vi "IV_Sweep_tool_Probe_Station_Resistance_2PP_2019_11_20.vi"() -> ()   [LabVIEW 2017]
doc: "I. Description:\nThis example demonstrates how to continuously acquire and generate data at the same time, synchronized with one another.\n\nII. Instructions for Running:\n1. Select the physical channel to correspond to where your signal is input on the DAQ device. Also, select the corresponding channel for where your signal is being generated.\n2. Enter the minimum and maximum voltage ranges.\nNote: For better accuracy try to match the input range to the expected voltage level of the measured signal.\n3. Set the sample rate of the acquisition.\nNote: The rate should be at least twice as fast as the maximum frequency component of the signal being acquired. \n6. Select the Rate for the generation\n7. Select what type of signal to generate and the amplitude.\nNote: This example requires two DMA channels to run. If your hardware does not support two DMA channels, you need to set the Data Transfer Mechanism property for the Analog Output Task to use \"Interrupts\". The Data Transfer Mechanism property is located in the DAQmx Channel Property hierarchy at:\n\nDAQmx Channel Property Node>>Analog Output>>General Properties>>Advanced>>Data Transfer and Memory>>Data Transfer Mechanism\n\nRefer to your device documentation to determine how many DMA channels are supported for your hardware.\n\nIII. Block Diagram Steps:\n1. Create an analog input voltage channel. Also, create an analog output voltage channel.\n2. Set the rate for the sample clock. Additionally, define the sample mode to be continuous. Also, set the sample clock rate for the signal generation.\n2a. Call the Get Terminal Name with Device Prefix VI. This will take a Task and a terminal and create a properly formatted device + terminal name to use as the source of the Trigger.\n3. Define the parameters for a Digital Edge Start Trigger. Set the Analog output to trigger off the AI Start Trigger. This is an internal trigger signal.\n4. Use the Basic Function Generator VI to create the signal to be generated.\n5. Call the Start VI to arm the two functions. Make sure the analog output is armed before the analog input. This will ensure both will start at the same time.\n6. Read the waveform data in a loop until the user hits the stop button or an error occurs. The Is Task Done? VI is used to check for errors in the Analog Output Task.\n7. Call the Clear VI to Clear the Task\n8. Use the popup dialog box to display an error if any.\n\nIV. I/O Connections Overview:\nMake sure your signal input/output terminals match the Physical Channel I/O controls."
uses:
  <vilib>/Utility/error.llb/DialogType.ctl
  <vilib>/DAQmx/write.llb/DAQmx Write (Analog 2D DBL NChan NSamp).vi
  <vilib>/DAQmx/read.llb/DAQmx Read (Analog 1D DBL NChan 1Samp).vi
  <vilib>/DAQmx/write.llb/DAQmx Write (Analog DBL 1Chan 1Samp).vi
  <vilib>/DAQmx/read.llb/DAQmx Read (Analog DBL 1Chan 1Samp).vi
  <vilib>/Analysis/baseanly.llb/Mean (DBL).vi
  <vilib>/DAQmx/write.llb/DAQmx Write (Analog 1D DBL NChan 1Samp).vi
  <vilib>/DAQmx/create/channels.llb/DAQmx Create Channel (AO-Voltage-Basic).vi
  <vilib>/DAQmx/create/channels.llb/DAQmx Create Channel (AI-Voltage-Basic).vi
  <vilib>/DAQmx/configure/timing.llb/DAQmx Timing (Sample Clock).vi
  <vilib>/DAQmx/configure/trigger.llb/DAQmx Start Trigger (Digital Edge).vi
  <vilib>/DAQmx/miscellaneous.llb/DAQmx Fill In Error Info.vi
  <vilib>/Utility/file.llb/Write To Spreadsheet File (DBL).vi
  <vilib>/Utility/file.llb/Write To Spreadsheet File (string).vi
  pid/pid.llb/PID (DBL).vi
  pid/pid.llb/PID Output Rate Limiter (DBL).vi
  <vilib>/ptbypt/NI_PtbyPt.lvlib
  <resource>/objmgr/daqmx.rc
  <vilib>/Analysis/NI_AALBase.lvlib
  <vilib>/Analysis/NI_AALPro.lvlib
panel:
  in  "Take a Screenshot":bool=TRUE
  in  "Current Amplifier\n1/Gain  (A/V)":dbl=-1e-11 format="%#_13g"
  out "Date and Time":string
  out "Bias Sweep 2":dbl[](graph)
  out "Array":dbl[](array[numeric])
  out "intercept":dbl
  out "Resistance (Ohms) \n[AI 1 must be connected to Vout (AO 0)]\n[Ensure current amplifier gain is correct]":dbl
  out "RTD-IV":cluster{dbl[], dbl[]}(graph)
  in  "Bias Offset Correct":dbl
  out "Bias Sweep":dbl[](graph)
  out "element":dbl
  out "mean":dbl format="%.6f"
  out "size(s)":i32
  out "Numeric":i32
  in  "PID":bool=TRUE caption="Step Z"
  in  "Tab Control":enum32{"PID Controller", "Tapping Controls"}(tab)=enum."Tapping Controls"
  in  "Proportional Gain":dbl=0.0001
  in  "Integral Gain":dbl=1e-07
  in  "Differential Gain":dbl=1e-05
  in  "Setpoint":dbl=0.1
  in  "Piezo Delta rate":dbl=1000.0
  in  "Min Current":dbl=0.002
  in  "Max Current":dbl=10.2
  in  "Ramp Rate":dbl=20.0
  in  "Make Contact":i32=1200
  in  "Break Contact":i32=500
  in  "Step Length":i32=100
  in  "Step Max":dbl=0.3
  in  "Step Min":dbl=0.05
  out "Tapping Stop":bool
  out "Case":i32
  in  "Contact Cycles":i32
  in  "Tapping":bool caption="Step Z"
  out "x/y":dbl
  out "Waveform Chart":dbl(graph)
  in  "Analog Output 1":dbl(slide) min=-10.0 max=10.0 step=0.001 scale=-10.0..10.0
  in  "Manual Z":bool caption="Step Z"
  in  "Sweep Amplitude":dbl=10.0
  in  "Stop Sweep":bool
  out "Connections 2":string="AI0=Current\nAI1=Bias\nAI2=dI/dV\nAI3=d2I/dV2\nAI4=X-Axis\nAI5=Z-Axis\n"
  out "Connections":string="AO0=Bias\nAO1=Z-axis\nAO2=X-Axis\nAO3=NA"
  out "Save Indicator":bool
  in  "Z-Direction":bool caption="Step Z"
  in  "Update Bias":bool
  in  "Save IV":bool
  in  "Save Decay":bool
  in  "Sweep Bias":bool
  in  "Step Z":bool
  in  "Comments and Experimental Notes":string="Molecule=TP4\nGain=10nA\nBias Gain=div/1\nSweep Freq.=0.0008Hz\nRef. Bias=4mV\nRef. Freq=2.977kHz\nGain LIA1=2mV\nTC LIA1=1s\nGain LIA2=5mV\nTC LIA2=1s\nLIA1=EGG\nLIA2=SRS\nEGG is driving(possible 5mV offset)"
  in  "Filenumber":i32
  in  "DATA Filename":string="Data_"
  in  "Data Directory":path=path "E:/Research/Data"
  out "Current Decay":cluster{dbl[], dbl[]}(graph)
  out "d2I/dV2":cluster{dbl[], dbl[]}(graph)
  out "dI/dV":cluster{dbl[], dbl[]}(graph)
  out "IV":cluster{dbl[], dbl[]}(graph)
  in  "# Samples":i32=2000
  in  "Frequency (Hz)":dbl=0.1
  out "Measurement 2":cluster{i32, dbl, dbl[]}(graph) caption="Measurement"
  out "Actual Update Generation Rate 2":dbl=5000.0 caption="Actual Update Generation Rate" format="%0.2f"
  in  "stop 3":bool
  in  "Bias":dbl caption="Bias Start Point" step=0.1 format="%_3g"
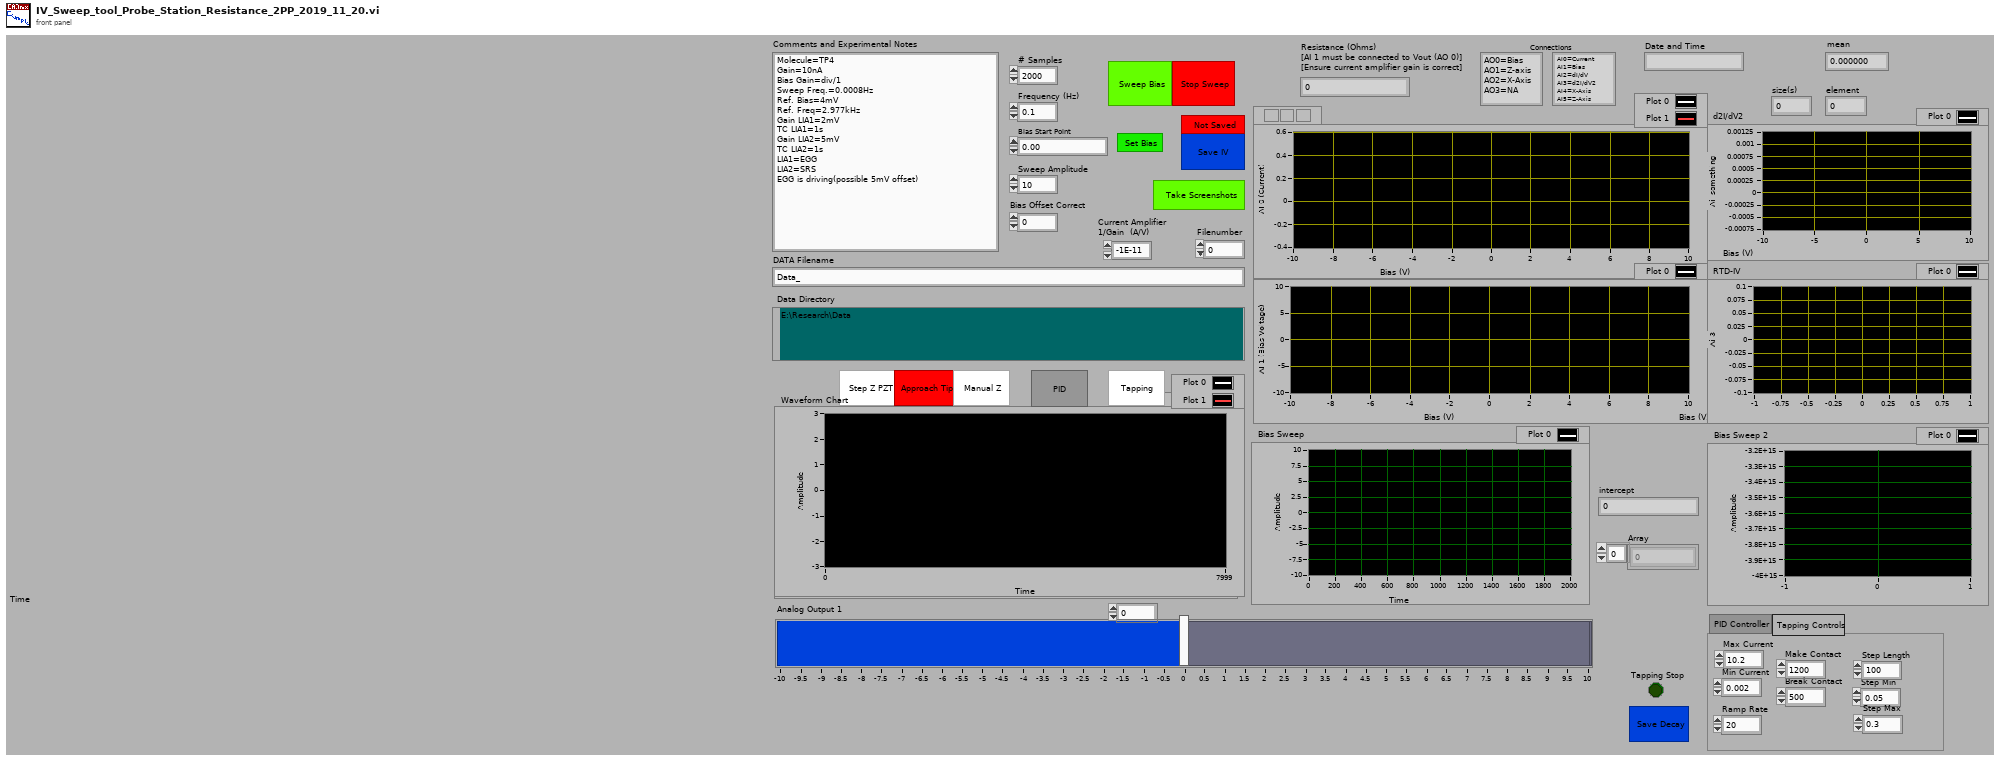
[diagram p1: front panel]
types:
  T1 = enum16{"open", "replace", "create", "open or create", "replace or create", "replace or create with confirmation"}
  T2 = typedef "DialogType.ctl" = u16
  T3 = cluster{"Proportional Gain":dbl, "Integral Gain ":dbl, "Differential Gain":dbl}
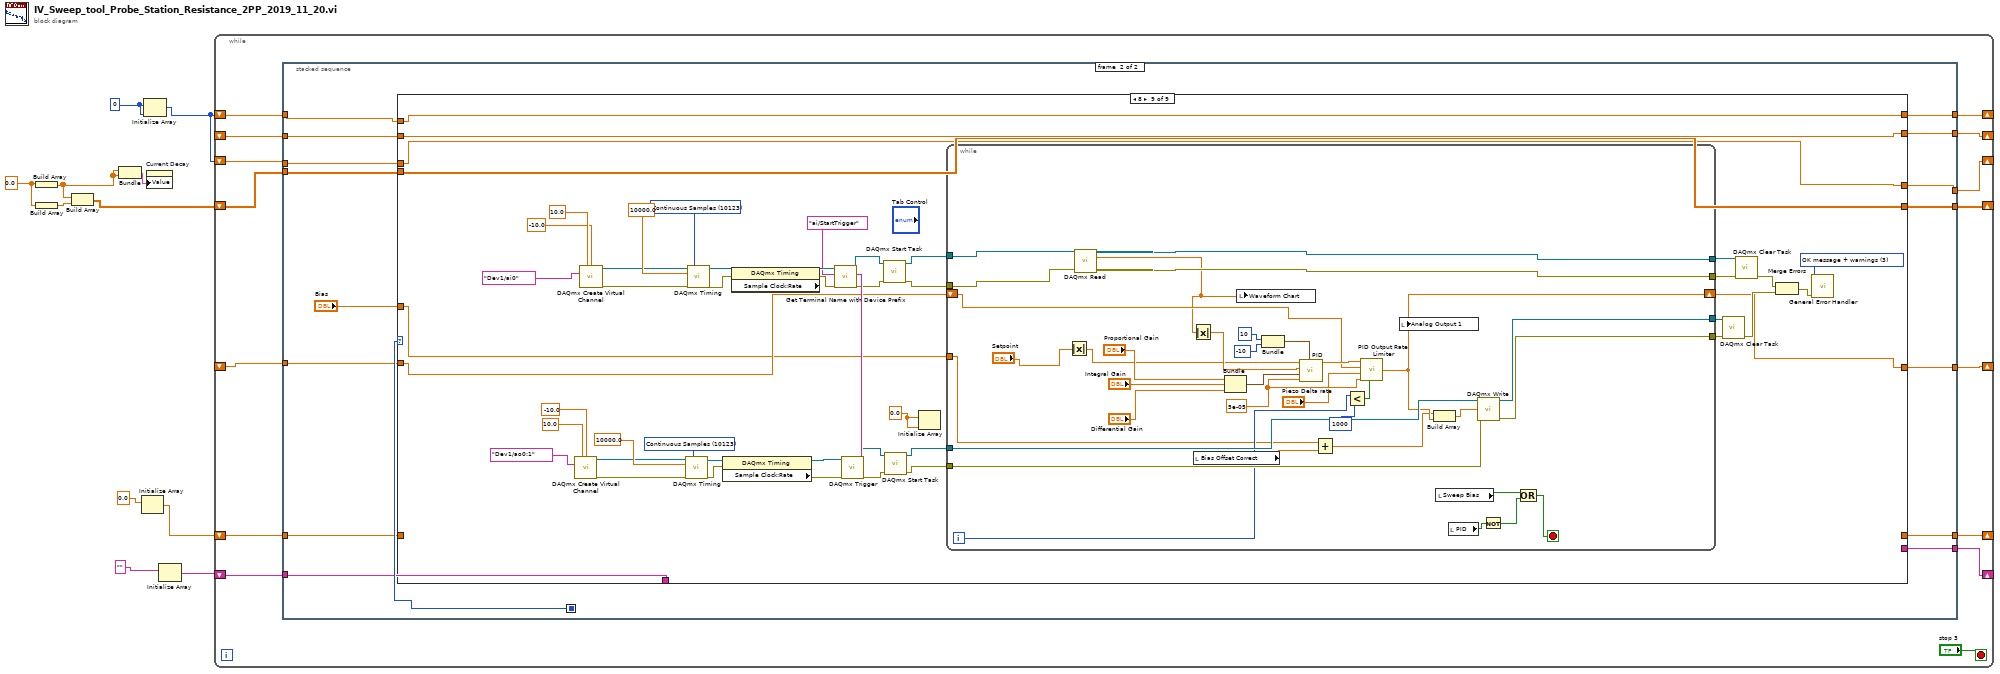
[diagram p0: block diagram]
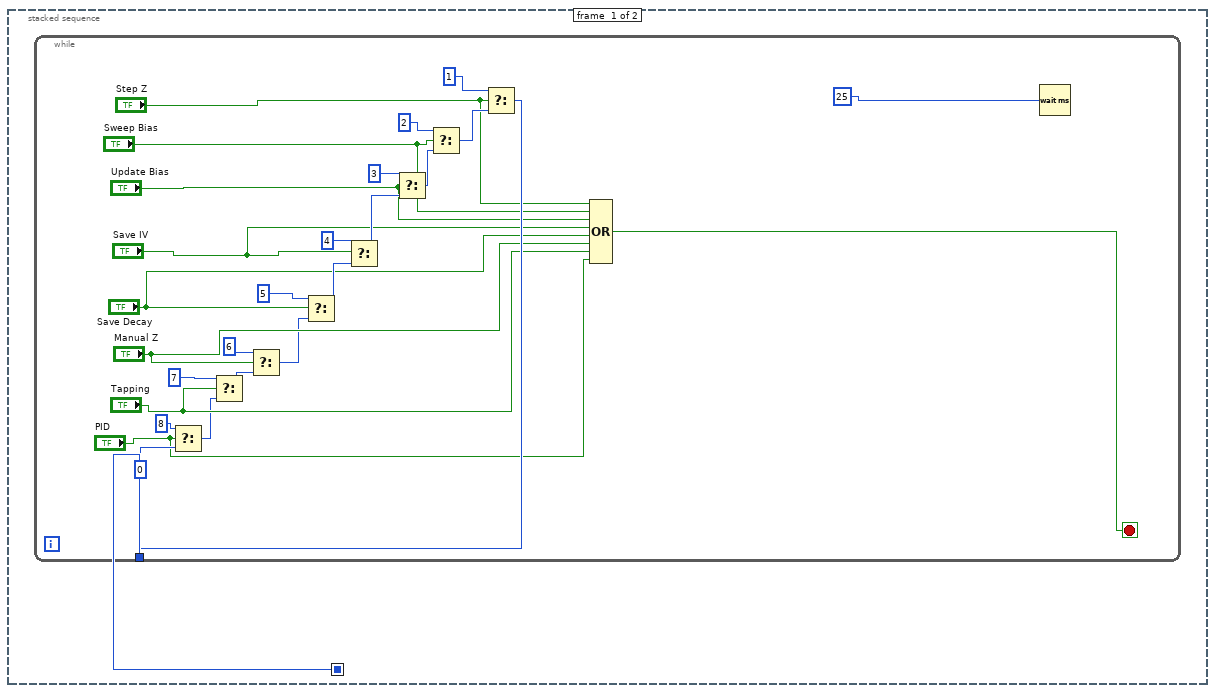
[diagram p2: hidden frame]
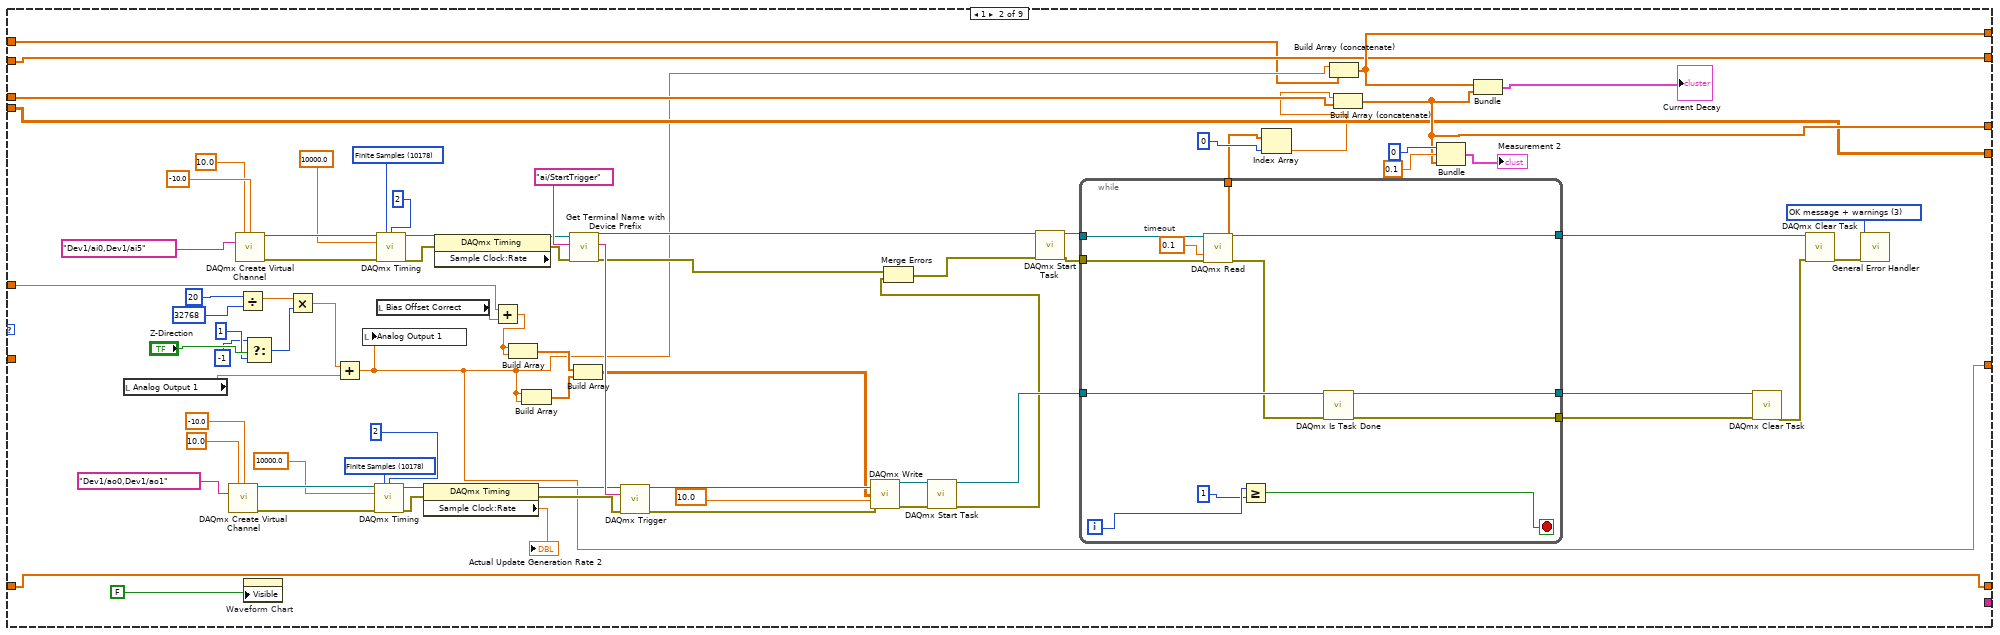
[diagram p4: hidden frame]
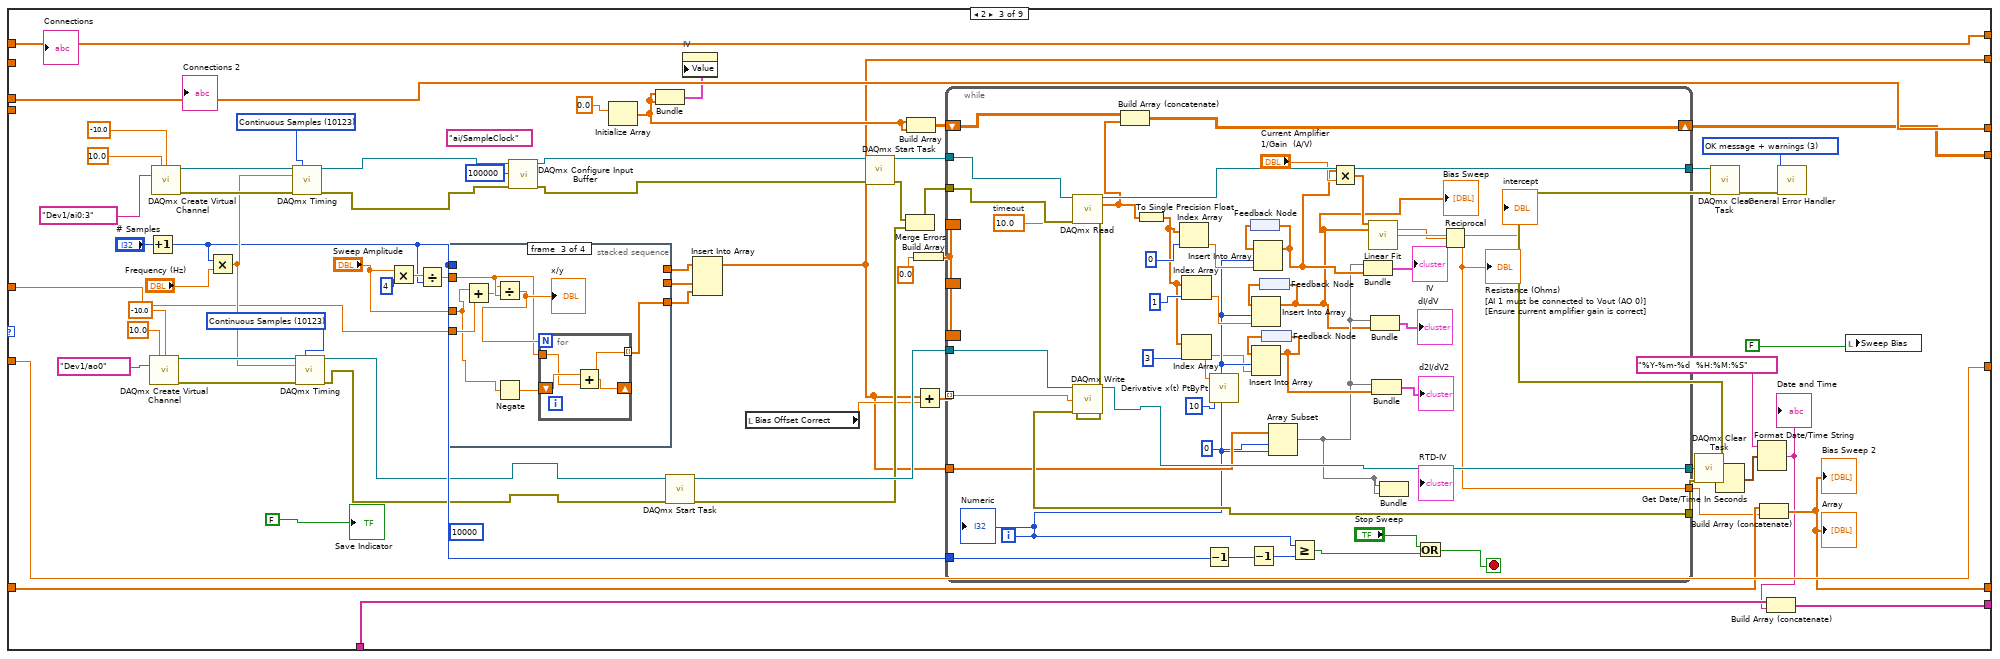
[diagram p5: hidden frame]
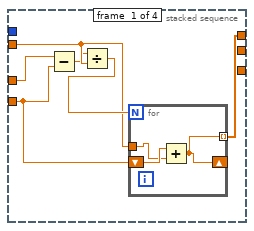
[diagram p6: hidden frame]
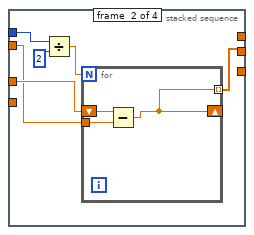
[diagram p7: hidden frame]
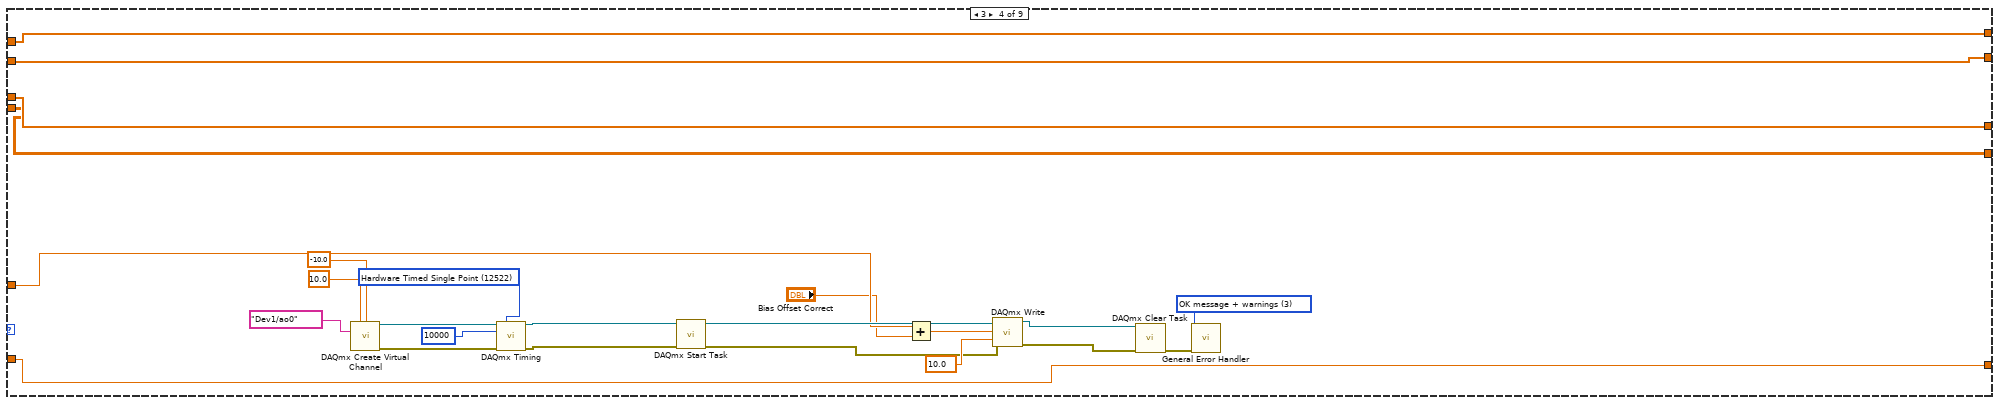
[diagram p9: hidden frame]
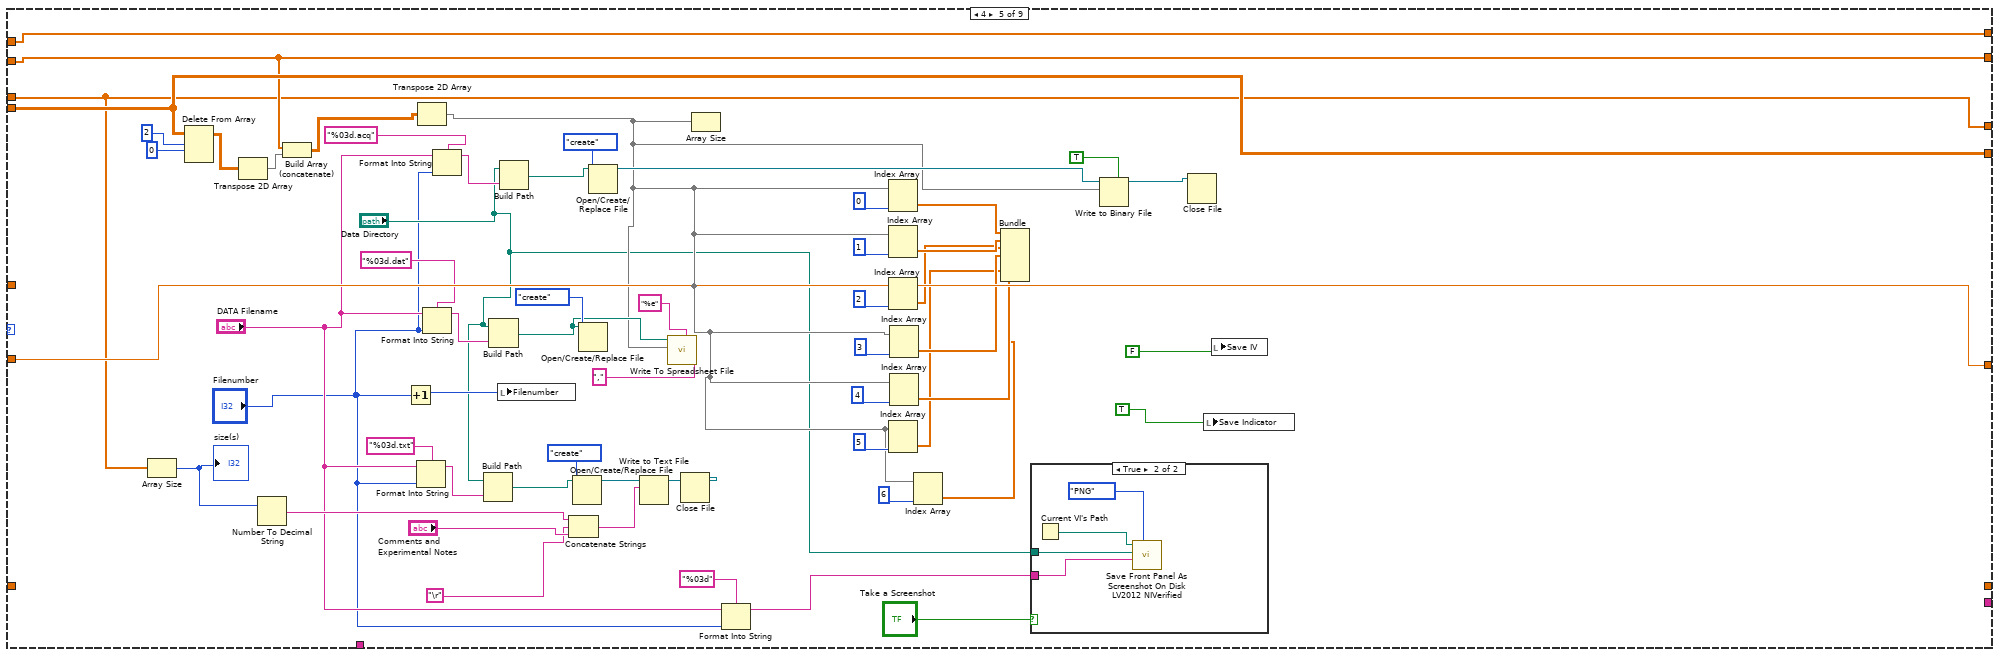
[diagram p10: hidden frame]
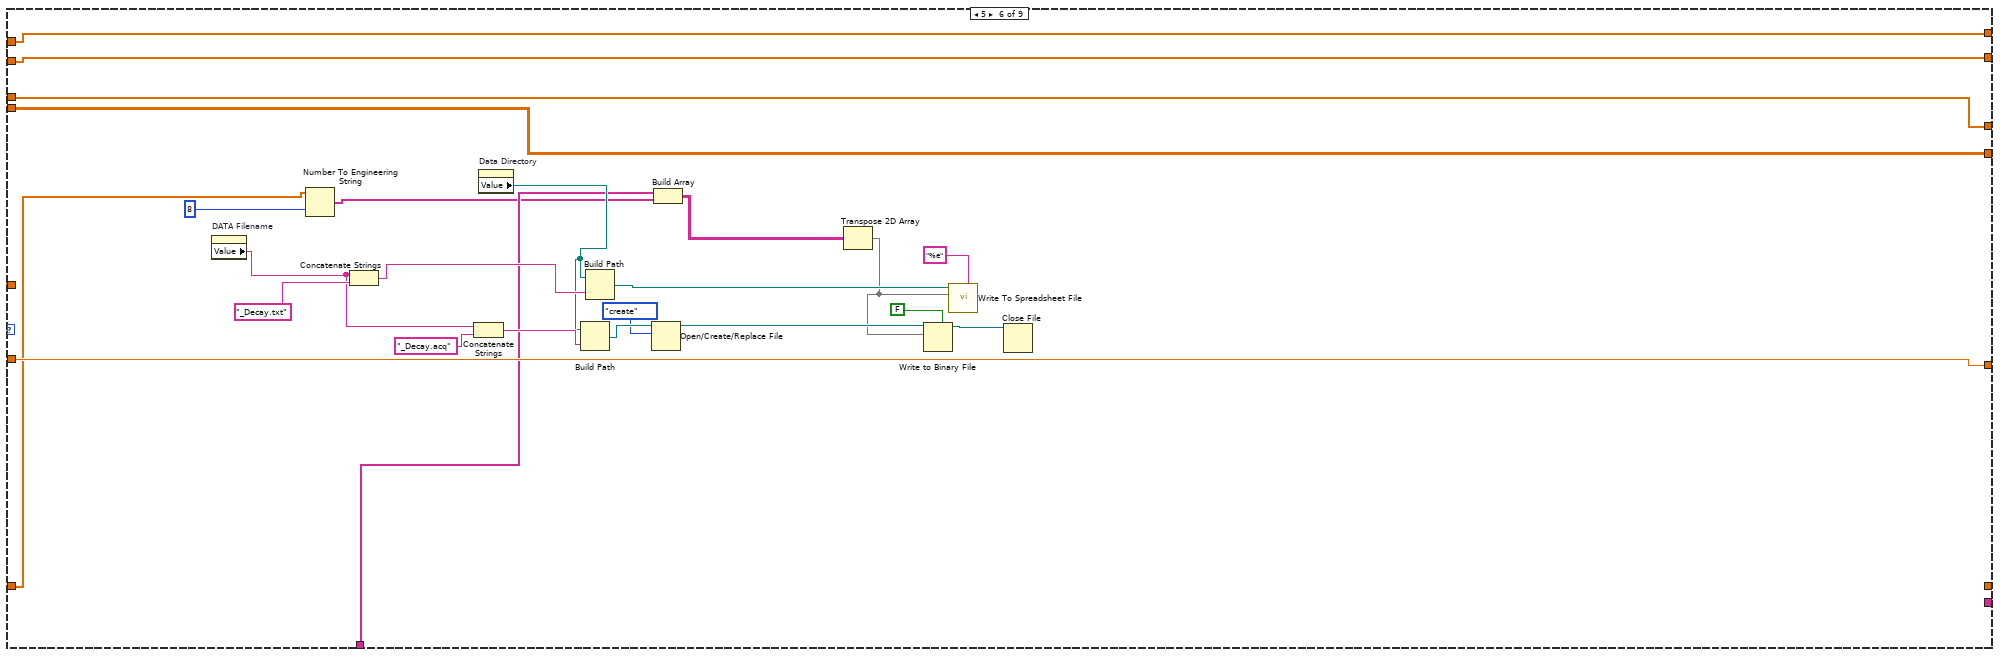
[diagram p12: hidden frame]
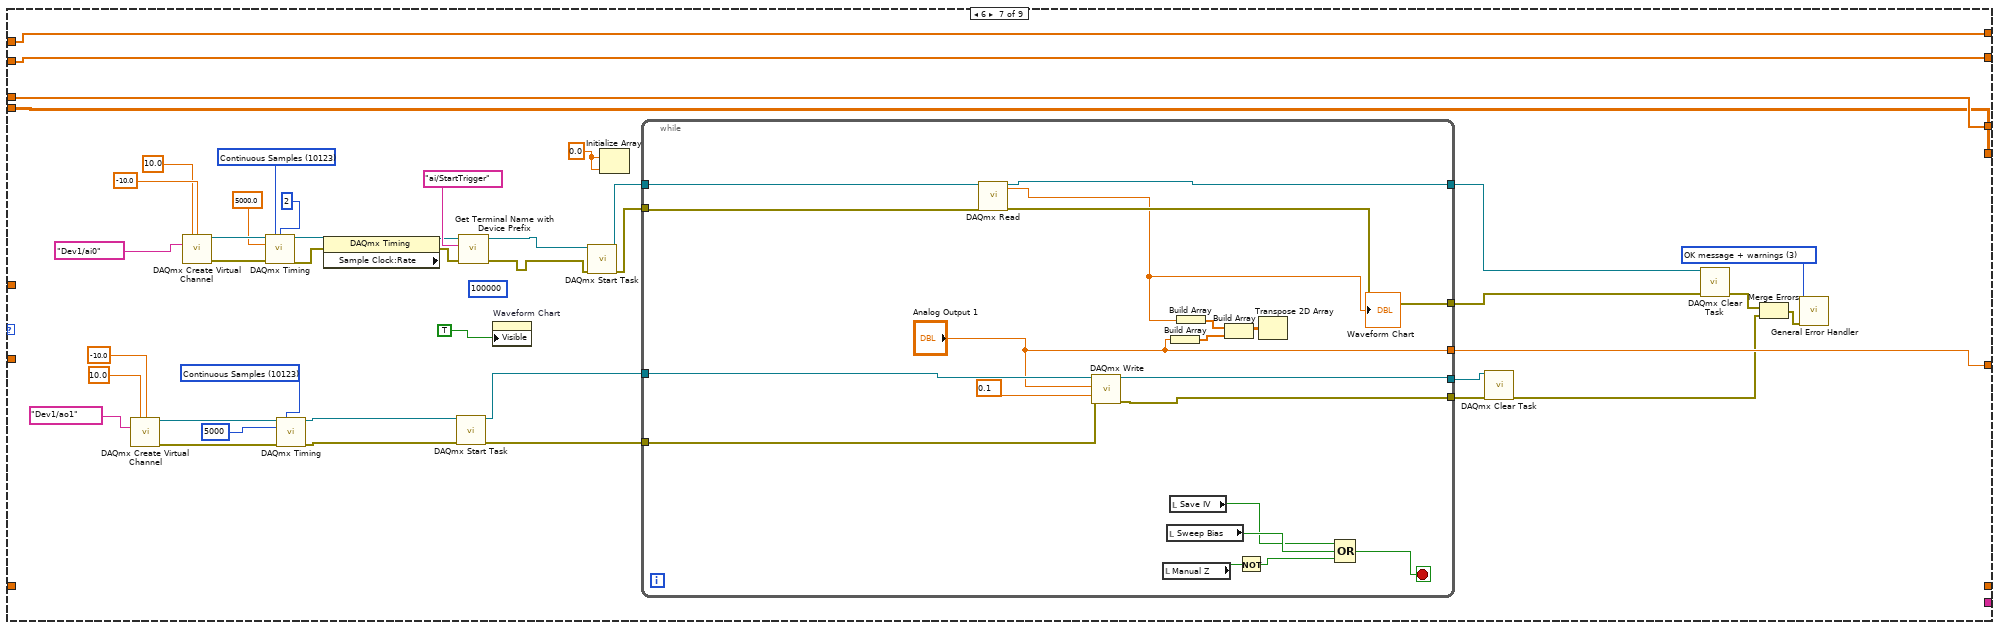
[diagram p13: hidden frame]
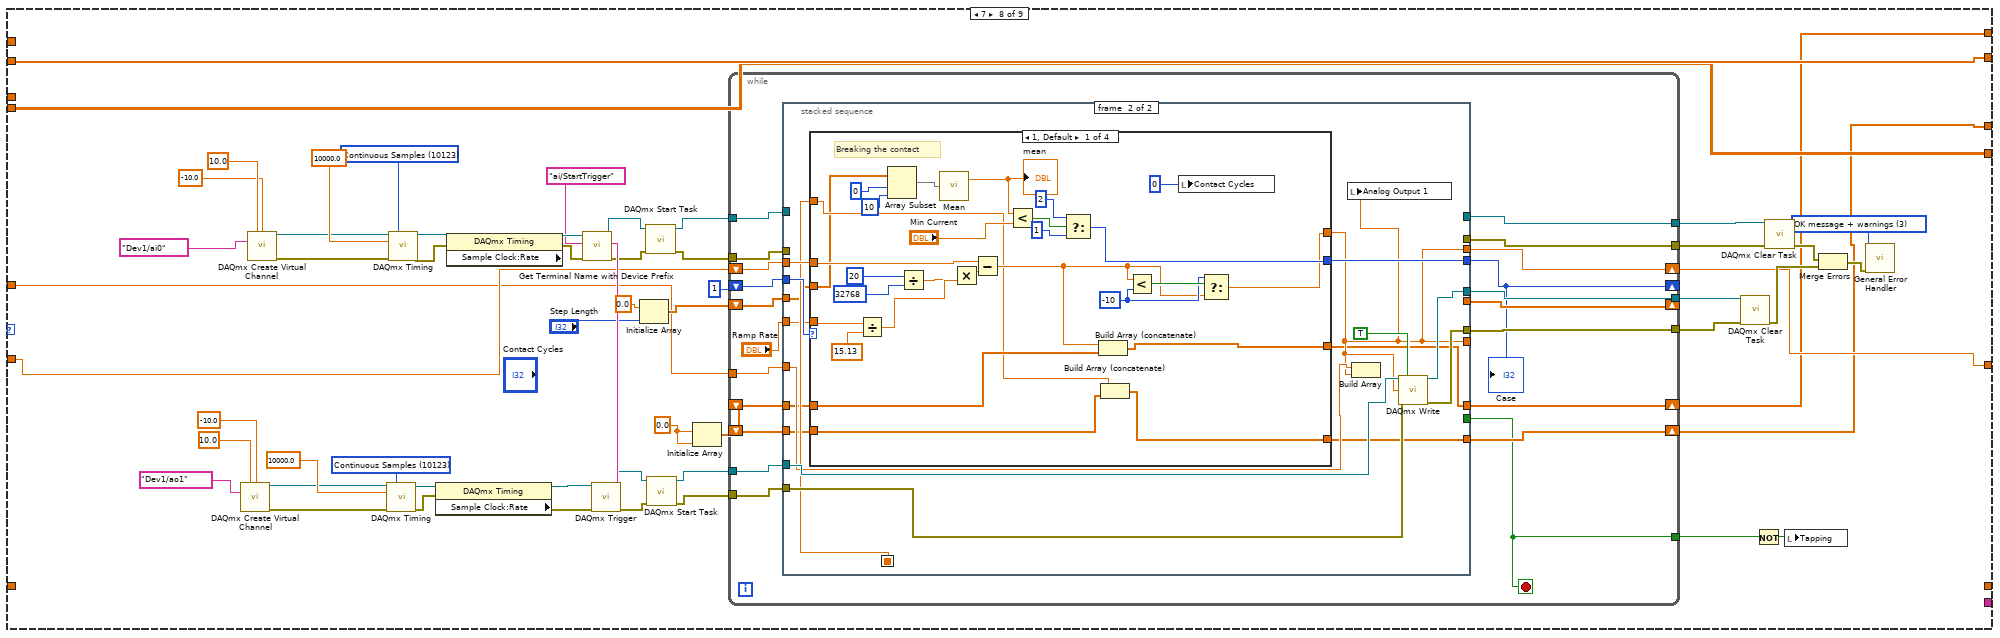
[diagram p14: hidden frame]
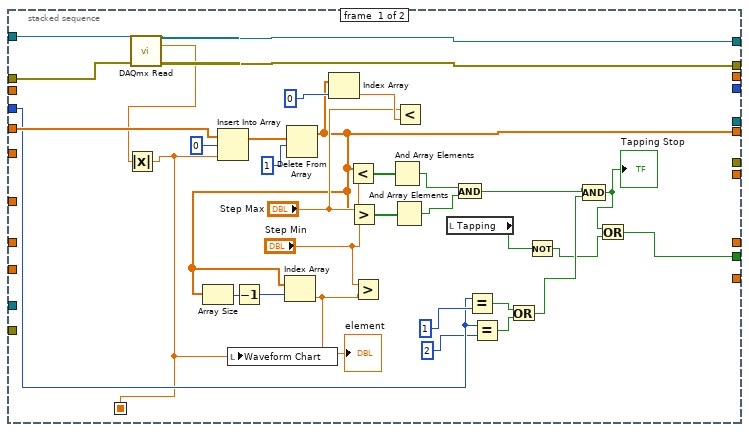
[diagram p15: hidden frame]
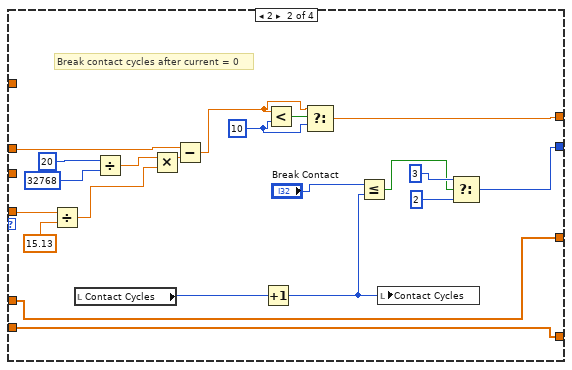
[diagram p16: hidden frame]
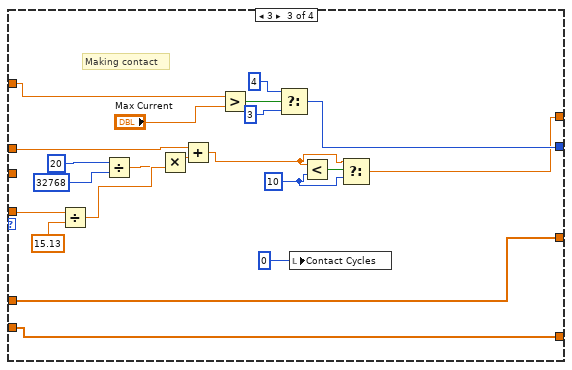
[diagram p17: hidden frame]
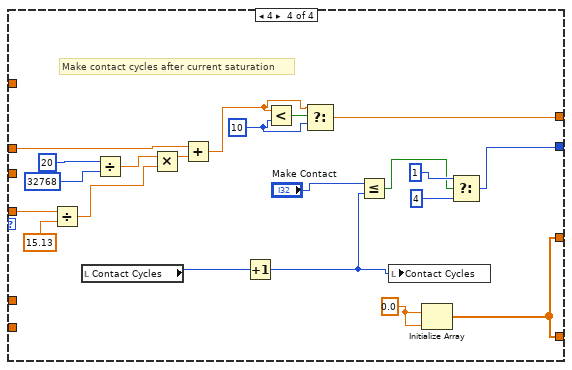
[diagram p18: hidden frame]
diagram:
  w6 = 0
  w11 = 0.0
  n1 = Build Array(w11) -> (w8:dbl[])
  n2 = Build Array(w11) -> (w10:dbl[])
  n3 = Build Array(w8, w10) -> (w9:dbl[][])
  n4 = Bundle(w8, w8) -> (w7:cluster{dbl[], dbl[]})  [unwired: 1 in]
  n5 = Initialize Array(0.0) -> (w3:dbl[])  [unwired: 1 in]
  n6 = Initialize Array(w6, w6) -> (w5:i32[])
  n7 = property on="Current Decay" class="XYGraph (strict)"("Value"=w7) -> ()  [unwired: 2 in, 2 out]
  n8 = Initialize Array("") -> (w1:string[])  [unwired: 1 in]
  n9 = while {
    shift-right: [w24] -> _
    shift-left: w5 -> [w25]
    shift-right: [w22] -> _
    shift-left: w5 -> [w23]
    shift-right: [w20] -> _
    shift-left: _ -> [w21]
    shift-right: [w18] -> _
    shift-left: w9 -> [w19]
    shift-right: [w16] -> _
    shift-left: _ -> [w17]
    shift-right: [w15] -> _
    shift-left: w3 -> [w14]
    shift-right: [w12] -> _
    shift-left: w1 -> [w13]
    stop <- "stop 3" stop-if-true
    n10 = stacked-sequence {
      seq-local: [w27 _] -> [_ w70]
      tunnel: w25 -> [_ w69]
      tunnel: [_ w68] -> w24
      tunnel: w23 -> [_ w66]
      tunnel: [_ w65] -> w22
      tunnel: w21 -> [_ w64]
      tunnel: [_ w59] -> w20
      tunnel: w19 -> [_ w63]
      tunnel: [_ w62] -> w18
      tunnel: w17 -> [_ w61]
      tunnel: [_ w60] -> w16
      tunnel: w14 -> [_ w58]
      tunnel: [_ w57] -> w15
      tunnel: w13 -> [_ w56]
      tunnel: [_ w55] -> w12
      frame #0 {
        n11 = while {
          tunnel: [w45] -> w27
          stop <- w44 stop-if-true
          n12 = Select(t=8, s="PID", f=0) -> (s? t:f=w31:i32)
          n13 = Select(t=7, s="Tapping", f=w31) -> (s? t:f=w33:i32)
          n14 = Select(t=6, s="Manual Z", f=w33) -> (s? t:f=w34:i32)
          n15 = Select(t=5, s="Save Decay", f=w34) -> (s? t:f=w50:i32)
          n16 = Select(t=4, s="Save IV", f=w50) -> (s? t:f=w49:i32)
          n17 = Select(t=3, s="Update Bias", f=w49) -> (s? t:f=w47:i32)
          n18 = Select(t=2, s="Sweep Bias", f=w47) -> (s? t:f=w54:i32)
          n19 = Select(t=1, s="Step Z", f=w54) -> (s? t:f=w45:i32)
          n20 = Compound Arithmetic op=OR("Step Z", "Sweep Bias", "Update Bias", "Save IV", "Save Decay", "Manual Z", "Tapping", "PID") -> (w44:bool)
          n21 = Wait (ms)(milliseconds to wait=25) -> ()  [unwired: 1 out]
        }
      }
      frame #1 {
        n22 = case shown="8" w70 {
          tunnel: w69 -> [w77 w85 w214 w310 w336 w393 w453 _ w693]
          tunnel: [w77 w98 w214 w310 w336 w393 w453 w479 w693] -> w68
          tunnel: "Bias" -> [_ w81 w199 w304 _ _ _ w485 w692]
          tunnel: w66 -> [w76 w82 w211 w311 w380 w409 w455 _ w694]
          tunnel: [w76 w99 w211 w311 w380 w409 w455 w480 w694] -> w65
          tunnel: w64 -> [w75 _ w210 w309 w379 w410 _ w486 w701]
          tunnel: [w75 w83 w210 w309 w379 w410 w424 w481 w698] -> w59
          tunnel: w63 -> [w74 w96 _ w307 w362 w411 w452 w483 w699]
          tunnel: [w74 w96 w191 w307 w362 w411 w452 w483 w699] -> w62
          tunnel: [w73 w91 w174 w306 w360 w394 w454 w484 w700] -> w60
          tunnel: w61 -> [w73 w91 _ w306 w360 w394 w454 w484 w700]
          tunnel: w58 -> [w72 w78 w173 _ _ w391 _ _ _]
          tunnel: [w72 w78 w171 _ _ _ _ _ _] -> w57
          tunnel: w56 -> [w71 _ w170 _ _ w392 _ _ _]
          tunnel: [w71 _ w169 _ _ _ _ _ _] -> w55
          frame 0, Default {
          }
          frame 1 {
            w133 = T2 3 items=["no dialog", "OK message", "continue or stop message", "OK message + warnings", "continue/stop + warnings"] ("type of dialog (OK msg:1)")
            w145 = 10178 items=["Finite Samples"=10178, "Continuous Samples"=10123] ("sample mode")
            w150 = 10178 items=["Finite Samples"=10178, "Continuous Samples"=10123] ("sample mode")
            n23 = local read "Analog Output 1"() -> (w86:dbl)
            n24 = call-poly <vilib>:"DAQmx Create Virtual Channel.vi"("maximum value"=10.0 ("maximum value 2"), "minimum value"=-10.0 ("minimum value 2"), "physical channels"=tag "Dev1/ao0,Dev1/ao1" ("physical channels 2")) -> ("task out"=w144:refnum<k21>, "error out"=w143:errorcluster)  [unwired: 11 in]
            n25 = call-poly <vilib>:"DAQmx Create Virtual Channel.vi"("maximum value"=10.0 ("Maximum Value 2"), "minimum value"=-10.0 ("Minimum Value 2"), "physical channels"=tag "Dev1/ai0,Dev1/ai5" ("Physical Channel 2")) -> ("task out"=w148:refnum<k21>, "error out"=w149:errorcluster)  [unwired: 11 in]
            n26 = Divide(x=20, y=32768) -> (x/y=w95:dbl)
            n27 = property on="Waveform Chart" class="WFChart (strict)"("Visible"=FALSE) -> ()  [unwired: 2 in, 2 out]
            n28 = Select(t=-1 ("f"), s="Z-Direction", f=1) -> (s? t:f=w93:i32)
            n29 = Multiply(x=w95, y=w93) -> (x*y=w94:dbl)
            n30 = Add(x=w94, y=w86) -> (x+y=w83:dbl)
            n31 = local write "Analog Output 1"(w83) -> ()
            n32 = call-poly <vilib>:"DAQmx Timing.vi"("task/channels in"=w144, "sample mode"=w145, "samples per channel"=2, "rate"=10000.0 ("rate 2"), "error in"=w143) -> ("task out"=w128:refnum<k21>, "error out"=w127:errorcluster)  [unwired: 9 in]
            n33 = call-poly <vilib>:"DAQmx Timing.vi"("task/channels in"=w148, "sample mode"=w150, "samples per channel"=2, "rate"=10000.0 ("Rate 2"), "error in"=w149) -> ("task out"=w122:refnum<k21>, "error out"=w121:errorcluster)  [unwired: 9 in]
            n34 = local read "Bias Offset Correct"() -> (w80:dbl)
            n35 = property class="DAQmx Timing"(reference=w128, error in=w127) -> (reference out=w129:refnum<k21>, error out=w126:errorcluster, "Sample Clock:Rate"=→"Actual Update Generation Rate 2":dbl)
            n36 = property class="DAQmx Timing" props=["Sample Clock:Rate"](reference=w122, error in=w121) -> (reference out=w120:refnum<k21>, error out=w119:errorcluster)  [unwired: 1 out]
            n37 = Add(x=w81, y=w80) -> (x+y=w79:dbl)
            n38 = Build Array(w79, w79) -> (w106:dbl[])
            n39 = Build Array(w83, w83) -> (w105:dbl[])
            n40 = call "Get Terminal Name with Device Prefix.vi"("error in (no error)"=w119, "Local Terminal Name"="ai/StartTrigger" ("terminal"), "task/channels in"=w120) -> ("error out"=w125:errorcluster, "Terminal Name with Device Prefix"=w130:tag, "task out"=w110:refnum<k21>)  [unwired: 6 in]
            n41 = Build Array(w106, w105) -> (w104:dbl[][])
            n42 = call-poly <vilib>:"DAQmx Trigger.vi"("task/channels in"=w129, "source"=w130, "error in"=w126) -> ("task out"=w135:refnum<k21>, "error out"=w136:errorcluster)  [unwired: 11 in]
            n43 = call-poly <vilib>:"DAQmx Write.vi"("task/channels in"=w135, "data"=w104, "timeout"=10.0 ("Wirite Timeout"), "error in"=w136) -> ("task out"=w138:refnum<k21>, "error out"=w137:errorcluster)  [unwired: 9 in, 1 out]
            n44 = call <vilib>:"DAQmx Start Task.vi"("task/channels in"=w138, "error in"=w137) -> ("task out"=w142:refnum<k21>, "error out"=w124:errorcluster)  [unwired: 12 in]
            n45 = Merge Errors(w125, w124) -> (w112:errorcluster)
            n46 = call <vilib>:"DAQmx Start Task.vi"("task/channels in"=w110, "error in"=w112) -> ("task out"=w109:refnum<k21>, "error out"=w111:errorcluster)  [unwired: 12 in]
            n47 = while {
              tunnel: [w165] -> w151
              tunnel: w142 -> [w164]
              tunnel: [w163] -> w141
              tunnel: w109 -> [w154]
              tunnel: [w162] -> w118
              tunnel: [w159] -> w102
              tunnel: w111 -> [w155]
              i -> [w158]
              stop <- w156 stop-if-true
              w161 = 0.1  # timeout
              n48 = call-poly <vilib>:"DAQmx Read.vi"("task/channels in"=w154, "timeout"=w161, "error in"=w155) -> ("task out"=w165:refnum<k21>, "data"=w159:dbl[], "error out"=w160:errorcluster)  [unwired: 10 in]
              n49 = Greater Or Equal?(x=w158, y=1) -> (x >= y?=w156:bool)
              n50 = call <vilib>:"DAQmx Is Task Done.vi"("task/channels in"=w164, "error in"=w160) -> ("task out"=w163:refnum<k21>, "error out"=w162:errorcluster)  [unwired: 11 in, 1 out]
            }
            n51 = Index Array(array=w102, index=0) -> (element=w84:dbl)
            n52 = Build Array (concatenate)(w83, w82) -> (w99:dbl[])
            n53 = Build Array (concatenate)(w84, w85) -> (w98:dbl[])
            n54 = Bundle(0, 0.1, w98) -> (→"Measurement 2":cluster{i32, dbl, dbl[]})  [unwired: 1 in]
            n55 = Bundle(w99, w98) -> (→"Current Decay":cluster{dbl[], dbl[]})  [unwired: 1 in]
            n56 = call <vilib>:"DAQmx Clear Task.vi"("task in"=w141, "error in"=w118) -> ("error out"=w117:errorcluster)  [unwired: 13 in]
            n57 = call <vilib>:"DAQmx Clear Task.vi"("task in"=w151, "error in"=w117) -> ("error out"=w116:errorcluster)  [unwired: 13 in]
            n58 = call <vilib>:"General Error Handler.vi"("type of dialog (OK msg:1)"=w133, "error in (no error)"=w116) -> ()  [unwired: 9 in, 5 out]
          }
          frame 2 {
            (unwired) 10000
            w208 = 10123 items=["Finite Samples"=10178, "Continuous Samples"=10123, "Hardware Timed Single Point"=12522] ("sample mode")
            w209 = 10123 items=["Finite Samples"=10178, "Continuous Samples"=10123, "Hardware Timed Single Point"=12522] ("sample mode")
            (unwired) "ai/SampleClock" ("terminal")
            w219 = T2 3 items=["no dialog", "OK message", "continue or stop message", "OK message + warnings", "continue/stop + warnings"] ("type of dialog (OK msg:1)")
            n59 = Increment(x="# Samples") -> (x+1=w189:i32)
            n60 = call-poly <vilib>:"DAQmx Create Virtual Channel.vi"("maximum value"=10.0, "minimum value"=-10.0, "physical channels"=tag "Dev1/ao0") -> ("task out"=w222:refnum<k21>, "error out"=w221:errorcluster)  [unwired: 11 in]
            n61 = call-poly <vilib>:"DAQmx Create Virtual Channel.vi"("maximum value"=10.0 ("Maximum Value"), "minimum value"=-10.0 ("Minimum Value"), "physical channels"=tag "Dev1/ai0:3" ("Physical Channel")) -> ("task out"=w226:refnum<k21>, "error out"=w227:errorcluster)  [unwired: 11 in]
            n62 = Multiply(x=w189, y="Frequency (Hz)") -> (x*y=w213:dbl)
            n63 = call-poly <vilib>:"DAQmx Timing.vi"("task/channels in"=w226, "sample mode"=w208, "rate"=w213, "error in"=w227) -> ("task out"=w183:refnum<k21>, "error out"=w181:errorcluster)  [unwired: 10 in]
            n64 = call-poly <vilib>:"DAQmx Timing.vi"("task/channels in"=w222, "sample mode"=w209, "rate"=w213, "error in"=w221) -> ("task out"=w178:refnum<k21>, "error out"=w177:errorcluster)  [unwired: 10 in]
            n65 = Multiply(x="Sweep Amplitude", y=4) -> (x*y=w197:dbl)
            n66 = Divide(x=w197, y=w189) -> (x/y=w196:dbl)
            n67 = stacked-sequence {
              tunnel: "Sweep Amplitude" -> [w280 w286 w294 _]
              tunnel: w199 -> [w278 _ w298 _]
              tunnel: w196 -> [w276 w285 w296 _]
              tunnel: [w277 _ _ _] -> w195
              tunnel: w189 -> [_ w289 _ _]
              tunnel: [_ w284 _ _] -> w194
              tunnel: [_ _ w297 _] -> w193
              frame #0 {
                n68 = Subtract(x=w280, y=w278) -> (x-y=w275:dbl)
                n69 = Divide(x=w275, y=w276) -> (x/y=w279:dbl)
                n70 = for {
                  N: w279 -> [_]
                  tunnel: w276 -> [w282]
                  shift-right: [w281] -> _
                  shift-left: w278 -> [w283]
                  tunnel: [w281] -> w277 mode=indexing
                  n71 = Add(x=w283, y=w282) -> (x+y=w281:dbl)
                }
              }
              frame #1 {
                n72 = Divide(x=w289, y=2) -> (x/y=w287:dbl)
                n73 = for {
                  N: w287 -> [_]
                  tunnel: w285 -> [w291]
                  shift-right: [w290] -> _
                  shift-left: w286 -> [w292]
                  tunnel: [w290] -> w284 mode=indexing
                  n74 = Subtract(x=w292, y=w291) -> (x-y=w290:dbl)
                }
              }
              frame #2 {
                n75 = Add(x=w294, y=w298) -> (x+y=w295:dbl)
                n76 = Divide(x=w295, y=w296) -> (x/y=w299:dbl)
                "x/y" <- w299
                n77 = Negate(x=w294) -> (-x=w293:dbl)
                n78 = for {
                  N: w299 -> [_]
                  tunnel: w296 -> [w301]
                  shift-right: [w300] -> _
                  shift-left: w293 -> [w302]
                  tunnel: [w300] -> w297 mode=indexing
                  n79 = Add(x=w302, y=w301) -> (x+y=w300:dbl)
                }
              }
              frame #3 {
              }
            }
            n80 = call <vilib>:"DAQmx Configure Input Buffer.vi"("task/channels in"=w183, "buffer size (in samples per channel)"=100000, "error in"=w181) -> ("task out"=w182:refnum<k21>, "error out"=w180:errorcluster)  [unwired: 11 in]
            n81 = Initialize Array(0.0) -> (w188:dbl[])  [unwired: 1 in]
            n82 = Bundle(w188, w188) -> (w187:cluster{dbl[], dbl[]})  [unwired: 1 in]
            n83 = call <vilib>:"DAQmx Start Task.vi"("task/channels in"=w178, "error in"=w177) -> ("task out"=w207:refnum<k21>, "error out"=w203:errorcluster)  [unwired: 12 in]
            n84 = property on="IV" class="XYGraph (strict)"("Value"=w187) -> ()  [unwired: 2 in, 2 out]
            n85 = Insert Into Array(array=w195, new element #1=w194, new element #2=w193) -> (w174:dbl[])  [unwired: 1 in]
            n86 = local read "Bias Offset Correct"() -> (w175:dbl)
            n87 = call <vilib>:"DAQmx Start Task.vi"("task/channels in"=w182, "error in"=w180) -> ("task out"=w205:refnum<k21>, "error out"=w204:errorcluster)  [unwired: 12 in]
            n88 = Merge Errors(w204, w203) -> (w206:errorcluster)
            n89 = Build Array(w188, w188) -> (w190:dbl[][])
            n90 = Build Array(0.0) -> (w185:dbl[])
            n91 = Add(x=w174, y=w175) -> (x+y=w176:dbl[])
            n92 = while {
              tunnel: [w266] -> w228
              tunnel: [w269] -> w220
              tunnel: [w268] -> w217
              tunnel: w189 -> [w244]
              tunnel: w176 -> [w249] mode=indexing
              tunnel: w207 -> [w271]
              tunnel: w205 -> [w274]
              tunnel: w206 -> [w273]
              shift-right: [w250] -> w191
              shift-left: w190 -> [w267]
              tunnel: w174 -> [w264]
              border: w185 -> [_]
              border: w185 -> [_]
              border: w185 -> [_]
              tunnel: [w236] -> w172
              i -> [w245]
              stop <- w246 stop-if-true
              w270 = 10.0  # timeout
              n93 = call-poly <vilib>:"DAQmx Read.vi"("task/channels in"=w274, "timeout"=w270, "error in"=w273) -> ("task out"=w266:refnum<k21>, "data"=w252:dbl[], "error out"=w272:errorcluster)  [unwired: 10 in]
              n94 = call-poly <vilib>:"DAQmx Write.vi"("task/channels in"=w271, "data"=w249, "error in"=w272) -> ("task out"=w269:refnum<k21>, "error out"=w268:errorcluster)  [unwired: 10 in, 1 out]
              n95 = Build Array (concatenate)(w267, w252) -> (w250:dbl[][])
              n96 = To Single Precision Float(number=w252) -> (single precision float=w251:sgl[])
              n97 = Index Array(array=w251, index=0) -> (element=w262:sgl)
              n98 = Index Array(array=w251, index=1) -> (element=w258:sgl)
              n99 = Index Array(array=w251, index=3) -> (element=w240:sgl)
              n100 = Decrement(x=w244) -> (x-1=w242:i32)
              n101 = call <vilib>:"Derivative x(t) PtByPt.vi"("dt"=10, "x"=w240) -> ()  [unwired: 2 in, 2 out]
              n102 = Decrement(x=w242) -> (x-1=w243:i32)
              n103 = feedback #1() -> (w261:dbl[])
              n104 = Insert Into Array(array=w261, index=w245, new element=w262) -> (w234:dbl[])
              n105 = feedback-in #1(w234) -> ()
              n106 = feedback #2() -> (w257:dbl[])
              n107 = Insert Into Array(array=w257, index=w245, new element=w258) -> (w231:dbl[])
              "Bias Sweep" <- w231
              n108 = feedback-in #2(w231) -> ()
              n109 = feedback #3() -> (w256:dbl[])
              n110 = Insert Into Array(array=w256, index=w245, new element=w240) -> (w239:dbl[])
              n111 = feedback-in #3(w239) -> ()
              n112 = Array Subset(array=w264, index=0, length=w245) -> (w232:dbl[])
              n113 = Greater Or Equal?(x=w245, y=w243) -> (x >= y?=w247:bool)
              n114 = Multiply(x=w234, y="Current Amplifier\n1/Gain  (A/V)") -> (x*y=w233:dbl[])
              n115 = Bundle(w232, w234) -> (→"IV":cluster{dbl[], dbl[]})  [unwired: 1 in]
              n116 = call <vilib>:"Linear Fit.vi"("Y"=w233, "X"=w231) -> ("slope"=w237:dbl, "intercept"=→"intercept":dbl)  [unwired: 9 in, 3 out]
              n117 = Bundle(w232, w231) -> (→"dI/dV":cluster{dbl[], dbl[]})  [unwired: 1 in]
              n118 = Bundle(w232, w239) -> (→"d2I/dV2":cluster{dbl[], dbl[]})  [unwired: 1 in]
              n119 = Bundle(w232, w232) -> ()  [unwired: 1 in, 1 out]
              n120 = Or(x="Stop Sweep", y=w247) -> (x .or. y?=w246:bool)
              n121 = Reciprocal(x=w237) -> (1/x=w236:dbl)
              "Resistance (Ohms) \n[AI 1 must be connected to Vout (AO 0)]\n[Ensure current amplifier gain is correct]" <- w236
              "Numeric" <- w245
            }
            n122 = call <vilib>:"DAQmx Clear Task.vi"("task in"=w220, "error in"=w217) -> ("error out"=w216:errorcluster)  [unwired: 13 in]
            n123 = call <vilib>:"DAQmx Clear Task.vi"("task in"=w228, "error in"=w216) -> ("error out"=w215:errorcluster)  [unwired: 13 in]
            n124 = Get Date/Time In Seconds() -> (seconds since 1Jan1904=w167:timestamp)
            n125 = Format Date/Time String(time format string (%c)="%Y-%m-%d  %H:%M:%S", seconds (now)=w167) -> (date/time string=w166:string)  [unwired: 1 in]
            "Date and Time" <- w166
            n126 = Build Array (concatenate)(w173, w172) -> (w171:dbl[])
            "Array" <- w171
            "Bias Sweep 2" <- w171
            n127 = Build Array (concatenate)(w170, w166) -> (w169:string[])
            n128 = call <vilib>:"General Error Handler.vi"("type of dialog (OK msg:1)"=w219, "error in (no error)"=w215) -> ()  [unwired: 9 in, 5 out]
            n129 = local write "Sweep Bias"(FALSE) -> ()
            "Save Indicator" <- FALSE
          }
          frame 3 {
            w315 = T2 3 items=["no dialog", "OK message", "continue or stop message", "OK message + warnings", "continue/stop + warnings"] ("type of dialog (OK msg:1)")
            w320 = 12522 items=["Finite Samples"=10178, "Continuous Samples"=10123, "Hardware Timed Single Point"=12522] ("sample mode")
            n130 = call-poly <vilib>:"DAQmx Create Virtual Channel.vi"("maximum value"=10.0 ("maximum value 2"), "minimum value"=-10.0 ("minimum value 2"), "physical channels"=tag "Dev1/ao0" ("physical channels 2")) -> ("task out"=w323:refnum<k21>, "error out"=w322:errorcluster)  [unwired: 11 in]
            n131 = call-poly <vilib>:"DAQmx Timing.vi"("task/channels in"=w323, "sample mode"=w320, "rate"=10000, "error in"=w322) -> ("task out"=w319:refnum<k21>, "error out"=w318:errorcluster)  [unwired: 10 in]
            n132 = call <vilib>:"DAQmx Start Task.vi"("task/channels in"=w319, "error in"=w318) -> ("task out"=w317:refnum<k21>, "error out"=w316:errorcluster)  [unwired: 12 in]
            n133 = Add(x=w304, y="Bias Offset Correct") -> (x+y=w305:dbl)
            n134 = call-poly <vilib>:"DAQmx Write.vi"("task/channels in"=w317, "data"=w305, "timeout"=10.0 ("Wirite Timeout"), "error in"=w316) -> ("task out"=w313:refnum<k21>, "error out"=w312:errorcluster)  [unwired: 9 in, 1 out]
            n135 = call <vilib>:"DAQmx Clear Task.vi"("task in"=w313, "error in"=w312) -> ("error out"=w314:errorcluster)  [unwired: 13 in]
            n136 = call <vilib>:"General Error Handler.vi"("type of dialog (OK msg:1)"=w315, "error in (no error)"=w314) -> ()  [unwired: 9 in, 5 out]
          }
          frame 4 {
            n137 = Array Size(array=w336) -> (size(s)=w335:i32)
            "size(s)" <- w335
            n138 = Delete From Array(array=w362, length=2, index (row)=0) -> (array with subset deleted=w359:dbl[][])  [unwired: 1 in, 1 out]
            n139 = Transpose 2D Array(2D array=w359) -> (transposed array=w358:dbl[][])
            n140 = Number To Decimal String(number=w335) -> (decimal integer string=w334:string)  [unwired: 1 in]
            n141 = Build Array (concatenate)(w360, w358) -> (w340:dbl[][])
            n142 = Increment(x="Filenumber") -> (x+1=w382:i32)
            n143 = Format Into String(format string="%03d.txt", initial string="DATA Filename", "Filenumber") -> (resulting string=w370:string)  [unwired: 1 in, 1 out]
            n144 = Transpose 2D Array(2D array=w340) -> (transposed array=w339:dbl[][])
            n145 = Format Into String(format string="%03d.dat", initial string="DATA Filename", "Filenumber") -> (resulting string=w384:string)  [unwired: 1 in, 1 out]
            n146 = Format Into String(format string="%03d.acq", initial string="DATA Filename", "Filenumber") -> (resulting string=w377:string)  [unwired: 1 in, 1 out]
            n147 = Build Path(base path="Data Directory", name or relative path=w370) -> (appended path=w368:path)
            n148 = Build Path(base path="Data Directory", name or relative path=w384) -> (appended path=w381:path)
            n149 = local write "Filenumber"(w382) -> ()
            n150 = Build Path(base path="Data Directory", name or relative path=w377) -> (appended path=w375:path)
            n151 = Concatenate Strings(w334, "\r", "Comments and Experimental Notes") -> (w356:string)
            n152 = Open/Create/Replace File(file path (use dialog)=w368, operation (0:open)=T1."create") -> (refnum out=w366:refnum<file>)  [unwired: 4 in, 2 out]
            n153 = Open/Create/Replace File(file path (use dialog)=w381, operation (0:open)=T1."create") -> ()  [unwired: 4 in, 3 out]
            n154 = Open/Create/Replace File(file path (use dialog)=w375, operation (0:open)=T1."create") -> (refnum out=w374:refnum<file>)  [unwired: 4 in, 2 out]
            n155 = Write to Text File(file (use dialog)=w366, text=w356) -> (refnum out=w365:refnum<file>)  [unwired: 2 in, 2 out]
            n156 = call-poly <vilib>:"Write To Spreadsheet File.vi"("delimiter (\\t)"=",", "format (%.3f)"="%e", "2D data"=w339, "file path (dialog if empty)"=w381) -> ()  [unwired: 4 in, 1 out]
            n157 = Close File(refnum=w365) -> ()  [unwired: 1 in, 2 out]
            n158 = Array Size(array=w339) -> ()  [unwired: 1 out]
            n159 = Format Into String(format string="%03d", initial string="DATA Filename", "Filenumber") -> (resulting string=w327:string)  [unwired: 1 in, 1 out]
            n160 = Index Array(array=w339, index (col)=0) -> (element=w348:dbl[])  [unwired: 1 in]
            n161 = Index Array(array=w339, index (col)=1) -> (element=w347:dbl[])  [unwired: 1 in]
            n162 = Index Array(array=w339, index (col)=2) -> (element=w346:dbl[])  [unwired: 1 in]
            n163 = Index Array(array=w339, index (col)=5) -> (element=w343:dbl[])  [unwired: 1 in]
            n164 = Index Array(array=w339, index (col)=3) -> (element=w345:dbl[])  [unwired: 1 in]
            n165 = Index Array(array=w339, index (col)=4) -> (element=w344:dbl[])  [unwired: 1 in]
            n166 = Index Array(array=w339, index (col)=6) -> (element=w342:dbl[])  [unwired: 1 in]
            n167 = Bundle(w348, w347, w346, w345, w344, w343, w342) -> ()  [unwired: 1 in, 1 out]
            n168 = case shown="True" "Take a Screenshot" {
              tunnel: "Data Directory" -> [_ w387]
              tunnel: w327 -> [_ w386]
              frame False {
              }
              frame True {
                n169 = Current VI's Path() -> (path=w385:path)
                n170 = call "Save Front Panel As Screenshot On Disk LV2012 NIVerified.vi"("Image Type"=enum16{"JPEG", "PNG", "BMP"}."PNG", "Image Name"=w386, "Image Folder"=w387, "VI path"=w385) -> ()  [unwired: 7 in, 1 out]
              }
            }
            n171 = Write to Binary File(file (use dialog)=w374, data=w339, 5:TRUE ("prepend array or string size? (T)")) -> (refnum out=w372:refnum<file>)  [unwired: 3 in, 2 out]
            n172 = Close File(refnum=w372) -> ()  [unwired: 1 in, 2 out]
            n173 = local write "Save Indicator"(TRUE) -> ()
            n174 = local write "Save IV"(FALSE) -> ()
          }
          frame 5 {
            n175 = property on="DATA Filename" class="Str"() -> ("Value"=w404:string)  [unwired: 2 in, 2 out]
            n176 = Number To Engineering String(2:i16 8 ("width (-)"), 4:w391) -> (0:w390:string[])  [unwired: 2 in]
            n177 = Concatenate Strings(w404, "_Decay.txt") -> (w408:string)
            n178 = Concatenate Strings(w404, "_Decay.acq") -> (w402:string)
            n179 = property on="Data Directory" class="Path"() -> ("Value"=w401:path)  [unwired: 2 in, 2 out]
            n180 = Build Path(base path=w401, name or relative path=w402) -> (appended path=w400:path)
            n181 = Build Path(base path=w401, name or relative path=w408) -> (appended path=w407:path)
            n182 = Open/Create/Replace File(file path (use dialog)=w400, operation (0:open)=T1."create") -> (refnum out=w406:refnum<file>)  [unwired: 4 in, 2 out]
            n183 = Build Array(w392, w390) -> (w397:string[][])
            n184 = Transpose 2D Array(2D array=w397) -> (transposed array=w396:string[][])
            n185 = Write to Binary File(file (use dialog)=w406, data=w396, 5:FALSE ("prepend array or string size? (T)")) -> (refnum out=w405:refnum<file>)  [unwired: 3 in, 2 out]
            n186 = call-poly <vilib>:"Write To Spreadsheet File.vi"("format (%s)"="%e", "2D data"=w396, "file path (dialog if empty)"=w407) -> ()  [unwired: 5 in, 1 out]
            n187 = Close File(refnum=w405) -> ()  [unwired: 1 in, 2 out]
          }
          frame 6 {
            (unwired) 100000
            w416 = 0.0
            w438 = 10123 items=["Finite Samples"=10178, "Continuous Samples"=10123] ("sample mode")
            w442 = T2 3 items=["no dialog", "OK message", "continue or stop message", "OK message + warnings", "continue/stop + warnings"] ("type of dialog (OK msg:1)")
            w446 = 10123 items=["Finite Samples"=10178, "Continuous Samples"=10123, "Hardware Timed Single Point"=12522] ("sample mode")
            n188 = call-poly <vilib>:"DAQmx Create Virtual Channel.vi"("maximum value"=10.0 ("maximum value 2"), "minimum value"=-10.0 ("minimum value 2"), "physical channels"=tag "Dev1/ao1" ("physical channels 2")) -> ("task out"=w448:refnum<k21>, "error out"=w447:errorcluster)  [unwired: 11 in]
            n189 = call-poly <vilib>:"DAQmx Create Virtual Channel.vi"("maximum value"=10.0 ("Maximum Value 2"), "minimum value"=-10.0 ("Minimum Value 2"), "physical channels"=tag "Dev1/ai0" ("Physical Channel 2")) -> ("task out"=w436:refnum<k21>, "error out"=w437:errorcluster)  [unwired: 11 in]
            n190 = call-poly <vilib>:"DAQmx Timing.vi"("task/channels in"=w436, "sample mode"=w438, "samples per channel"=2, "rate"=5000.0 ("Rate 2"), "error in"=w437) -> ("task out"=w432:refnum<k21>, "error out"=w431:errorcluster)  [unwired: 9 in]
            n191 = call-poly <vilib>:"DAQmx Timing.vi"("task/channels in"=w448, "sample mode"=w446, "rate"=5000, "error in"=w447) -> ("task out"=w445:refnum<k21>, "error out"=w444:errorcluster)  [unwired: 10 in]
            n192 = property class="DAQmx Timing" props=["Sample Clock:Rate"](reference=w432, error in=w431) -> (reference out=w430:refnum<k21>, error out=w429:errorcluster)  [unwired: 1 out]
            n193 = call <vilib>:"DAQmx Start Task.vi"("task/channels in"=w445, "error in"=w444) -> ("task out"=w443:refnum<k21>, "error out"=w425:errorcluster)  [unwired: 12 in]
            n194 = call "Get Terminal Name with Device Prefix.vi"("error in (no error)"=w429, "Local Terminal Name"="ai/StartTrigger" ("terminal"), "task/channels in"=w430) -> ("error out"=w413:errorcluster, "task out"=w414:refnum<k21>)  [unwired: 6 in, 1 out]
            n195 = property on="Waveform Chart" class="WFChart (strict)"("Visible"=TRUE) -> ()  [unwired: 2 in, 2 out]
            n196 = call <vilib>:"DAQmx Start Task.vi"("task/channels in"=w414, "error in"=w413) -> ("task out"=w423:refnum<k21>, "error out"=w427:errorcluster)  [unwired: 12 in]
            n197 = Initialize Array(w416, w416) -> ()  [unwired: 1 out]
            n198 = while {
              tunnel: w443 -> [w474]
              tunnel: w427 -> [w473]
              tunnel: w425 -> [w472]
              tunnel: ["Analog Output 1"] -> w424
              tunnel: w423 -> [w471]
              tunnel: [w470] -> w422
              tunnel: [w469] -> w421
              tunnel: [w468] -> w419
              tunnel: [w462] -> w417
              stop <- w459 stop-if-true
              n199 = call-poly <vilib>:"DAQmx Read.vi"("task/channels in"=w471, "error in"=w473) -> ("task out"=w462:refnum<k21>, "data"=w457:dbl, "error out"=w468:errorcluster)  [unwired: 11 in]
              "Waveform Chart" <- w457
              n200 = call-poly <vilib>:"DAQmx Write.vi"("task/channels in"=w474, "data"="Analog Output 1", "timeout"=0.1 ("Wirite Timeout"), "error in"=w472) -> ("task out"=w470:refnum<k21>, "error out"=w469:errorcluster)  [unwired: 9 in, 1 out]
              n201 = local read "Manual Z"() -> (w456:bool)
              n202 = local read "Sweep Bias"() -> (w460:bool)
              n203 = local read "Save IV"() -> (w458:bool)
              n204 = Build Array("Analog Output 1") -> (w466:dbl[])
              n205 = Build Array(w457) -> (w465:dbl[])
              n206 = Build Array(w465, w466) -> (w464:dbl[][])
              n207 = Not(x=w456) -> (.not. x?=w461:bool)
              n208 = Transpose 2D Array(2D array=w464) -> ()  [unwired: 1 out]
              n209 = Compound Arithmetic op=OR(w458, w460, w461) -> (w459:bool)
            }
            n210 = call <vilib>:"DAQmx Clear Task.vi"("task in"=w422, "error in"=w421) -> ("error out"=w420:errorcluster)  [unwired: 13 in]
            n211 = call <vilib>:"DAQmx Clear Task.vi"("task in"=w417, "error in"=w419) -> ("error out"=w418:errorcluster)  [unwired: 13 in]
            n212 = Merge Errors(w418, w420) -> (w426:errorcluster)
            n213 = call <vilib>:"General Error Handler.vi"("type of dialog (OK msg:1)"=w442, "error in (no error)"=w426) -> ()  [unwired: 9 in, 5 out]
          }
          frame 7 {
            w478 = 0.0
            w499 = T2 3 items=["no dialog", "OK message", "continue or stop message", "OK message + warnings", "continue/stop + warnings"] ("type of dialog (OK msg:1)")
            w514 = 10123 items=["Finite Samples"=10178, "Continuous Samples"=10123] ("sample mode")
            w508 = 10123 items=["Finite Samples"=10178, "Continuous Samples"=10123] ("sample mode")
            n214 = call-poly <vilib>:"DAQmx Create Virtual Channel.vi"("maximum value"=10.0 ("maximum value 2"), "minimum value"=-10.0 ("minimum value 2"), "physical channels"=tag "Dev1/ao1" ("physical channels 2")) -> ("task out"=w515:refnum<k21>, "error out"=w516:errorcluster)  [unwired: 11 in]
            n215 = call-poly <vilib>:"DAQmx Create Virtual Channel.vi"("maximum value"=10.0 ("Maximum Value 2"), "minimum value"=-10.0 ("Minimum Value 2"), "physical channels"=tag "Dev1/ai0" ("Physical Channel 2")) -> ("task out"=w510:refnum<k21>, "error out"=w509:errorcluster)  [unwired: 11 in]
            n216 = call-poly <vilib>:"DAQmx Timing.vi"("task/channels in"=w515, "sample mode"=w514, "rate"=10000.0 ("rate 2"), "error in"=w516) -> ("task out"=w523:refnum<k21>, "error out"=w524:errorcluster)  [unwired: 10 in]
            n217 = call-poly <vilib>:"DAQmx Timing.vi"("task/channels in"=w510, "sample mode"=w508, "rate"=10000.0 ("Rate 2"), "error in"=w509) -> ("task out"=w526:refnum<k21>, "error out"=w527:errorcluster)  [unwired: 10 in]
            n218 = property class="DAQmx Timing" props=["Sample Clock:Rate"](reference=w523, error in=w524) -> (reference out=w522:refnum<k21>, error out=w525:errorcluster)  [unwired: 1 out]
            n219 = property class="DAQmx Timing" props=["Sample Clock:Rate"](reference=w526, error in=w527) -> (reference out=w528:refnum<k21>, error out=w529:errorcluster)  [unwired: 1 out]
            n220 = call "Get Terminal Name with Device Prefix.vi"("error in (no error)"=w529, "Local Terminal Name"="ai/StartTrigger" ("terminal"), "task/channels in"=w528) -> ("error out"=w497:errorcluster, "Terminal Name with Device Prefix"=w521:tag, "task out"=w495:refnum<k21>)  [unwired: 6 in]
            n221 = call-poly <vilib>:"DAQmx Trigger.vi"("task/channels in"=w522, "source"=w521, "error in"=w525) -> ("task out"=w490:refnum<k21>, "error out"=w487:errorcluster)  [unwired: 11 in]
            n222 = Initialize Array(0.0, "Step Length") -> (w493:dbl[])
            n223 = call <vilib>:"DAQmx Start Task.vi"("task/channels in"=w495, "error in"=w497) -> ("task out"=w494:refnum<k21>, "error out"=w496:errorcluster)  [unwired: 12 in]
            n224 = call <vilib>:"DAQmx Start Task.vi"("task/channels in"=w490, "error in"=w487) -> ("task out"=w489:refnum<k21>, "error out"=w488:errorcluster)  [unwired: 12 in]
            n225 = Initialize Array(w478, w478) -> (w477:dbl[])
            n226 = while {
              tunnel: w494 -> [w550]
              tunnel: w496 -> [w549]
              tunnel: w489 -> [w548]
              tunnel: w488 -> [w547]
              tunnel: [w546] -> w505
              tunnel: [w545] -> w504
              tunnel: [w544] -> w502
              tunnel: [w543] -> w500
              shift-right: [w541] -> _
              shift-left: w493 -> [w542]
              tunnel: w485 -> [w539]
              shift-right: [w538] -> _
              shift-left: 1 -> [w537]
              shift-right: [w536] -> w481
              shift-left: w486 -> [w540]
              shift-right: [w534] -> w480
              shift-left: w477 -> [w535]
              shift-right: [w532] -> w479
              shift-left: w477 -> [w533]
              tunnel: [w530] -> w476
              stop <- w530 stop-if-true
              n227 = stacked-sequence {
                seq-local: [w552 _] -> [_ w592]
                tunnel: w550 -> [w583 _]
                tunnel: w549 -> [w582 _]
                tunnel: w548 -> [_ w600]
                tunnel: w547 -> [_ w599]
                tunnel: [w580 _] -> w546
                tunnel: [w581 _] -> w545
                tunnel: [_ w597] -> w544
                tunnel: [_ w598] -> w543
                tunnel: w542 -> [w577 w584]
                tunnel: [w560 _] -> w541
                tunnel: [w553 _] -> w530
                tunnel: w540 -> [_ w596]
                tunnel: w539 -> [_ w595]
                tunnel: [_ w594] -> w538
                tunnel: w537 -> [w569 w593]
                tunnel: "Ramp Rate" -> [_ w591]
                tunnel: [_ w589] -> _
                tunnel: [_ w589] -> w536
                tunnel: w535 -> [_ w588]
                tunnel: [_ w587] -> w534
                tunnel: w533 -> [_ w586]
                tunnel: [_ w585] -> w532
                frame #0 {
                  n228 = call-poly <vilib>:"DAQmx Read.vi"("task/channels in"=w583, "error in"=w582) -> ("task out"=w580:refnum<k21>, "data"=w551:dbl, "error out"=w581:errorcluster)  [unwired: 11 in]
                  n229 = Absolute Value(x=w551) -> (abs(x)=w552:dbl)
                  n230 = Insert Into Array(array=w577, index=0, new element=w552) -> (w578:dbl[])
                  n231 = local write "Waveform Chart"(w552) -> ()
                  n232 = Delete From Array(array=w578, length=1) -> (array with subset deleted=w560:dbl[])  [unwired: 1 in, 1 out]
                  n233 = Array Size(array=w560) -> (size(s)=w570:i32)
                  n234 = Decrement(x=w570) -> (x-1=w561:i32)
                  n235 = Index Array(array=w560, index=w561) -> (element=w563:dbl)
                  "element" <- w563
                  n236 = Index Array(array=w560, index=0) -> (element=w565:dbl)
                  n237 = Less?(x=w560, y="Step Max") -> (x < y?=w575:bool[])
                  n238 = Greater?(x=w560, y="Step Min") -> (0:w574:bool[])
                  n239 = Greater?(x="Step Min", y=w563) -> ()  [unwired: 1 out]
                  n240 = And Array Elements(Boolean array=w575) -> (logical AND=w559:bool)
                  n241 = And Array Elements(Boolean array=w574) -> (logical AND=w558:bool)
                  n242 = Less?(x="Step Max", y=w565) -> ()  [unwired: 1 out]
                  n243 = local read "Tapping"() -> (w555:bool)
                  n244 = And(x=w559, y=w558) -> (x .and. y?=w573:bool)
                  n245 = Equal?(x=w569, y=1) -> (x = y?=w567:bool)
                  n246 = Equal?(x=w569, y=2) -> (x = y?=w566:bool)
                  n247 = Or(x=w567, y=w566) -> (x .or. y?=w557:bool)
                  n248 = Not(x=w555) -> (.not. x?=w554:bool)
                  n249 = Compound Arithmetic op=AND(w573, w557) -> (w556:bool)
                  "Tapping Stop" <- w556
                  n250 = Or(x=w556, y=w554) -> (x .or. y?=w553:bool)
                }
                frame #1 {
                  n251 = case shown="1, Default" w593 {
                    tunnel: [w608 w631 w652 w678] -> w589
                    tunnel: w596 -> [w621 w633 w663 w675]
                    tunnel: [w616 w632 w657 w674] -> w594
                    tunnel: w592 -> [w607 _ w662 _]
                    tunnel: w591 -> [w622 w636 w664 w673]
                    tunnel: w588 -> [w612 w630 w651 _]
                    tunnel: [w614 w630 w651 w671] -> w587
                    tunnel: w586 -> [w606 w629 w650 _]
                    tunnel: [w613 w629 w650 w671] -> w585
                    tunnel: w584 -> [w605 _ _ _]
                    frame 1, Default {
                      w610 = -10
                      # "Breaking the contact"
                      n252 = Divide(x=w622, y=15.13) -> (x/y=w626:dbl)
                      n253 = Array Subset(array=w605, index=0, length=10) -> (w602:dbl[])
                      n254 = Divide(x=20, y=32768) -> (x/y=w623:dbl)
                      n255 = call-poly <vilib>:"Mean.vi"("X"=w602) -> ("mean"=w601:dbl)  [unwired: 1 out]
                      "mean" <- w601
                      n256 = Multiply(x=w623, y=w626) -> (x*y=w628:dbl)
                      n257 = Subtract(x=w621, y=w628) -> (x-y=w609:dbl)
                      n258 = Less?(x=w601, y="Min Current") -> (x < y?=w619:bool)
                      n259 = Select(t=2, s=w619, f=1) -> (s? t:f=w616:i32)
                      n260 = Build Array (concatenate)(w609, w612) -> (w614:dbl[])
                      n261 = Build Array (concatenate)(w607, w606) -> (w613:dbl[])
                      n262 = Less?(x=w609, y=w610) -> (x < y?=w611:bool)
                      n263 = local write "Contact Cycles"(0) -> ()
                      n264 = Select(t=w610, s=w611, f=w609) -> (s? t:f=w608:dbl)
                    }
                    frame 2 {
                      w648 = 10
                      # "Break contact cycles after current = 0"
                      n265 = Divide(x=w636, y=15.13) -> (x/y=w644:dbl)
                      n266 = local read "Contact Cycles"() -> (w635:i32)
                      n267 = Divide(x=20, y=32768) -> (x/y=w637:dbl)
                      n268 = Multiply(x=w637, y=w644) -> (x*y=w646:dbl)
                      n269 = Subtract(x=w633, y=w646) -> (x-y=w638:dbl)
                      n270 = Increment(x=w635) -> (x+1=w634:i32)
                      n271 = Less?(x=w638, y=w648) -> (x < y?=w647:bool)
                      n272 = Select(t=w638, s=w647, f=w648) -> (s? t:f=w631:dbl)
                      n273 = Less Or Equal?(x="Break Contact", y=w634) -> (x <= y?=w641:bool)
                      n274 = local write "Contact Cycles"(w634) -> ()
                      n275 = Select(t=3, s=w641, f=2) -> (s? t:f=w632:i32)
                    }
                    frame 3 {
                      w655 = 10
                      # "Making contact"
                      n276 = Divide(x=w664, y=15.13) -> (x/y=w668:dbl)
                      n277 = Divide(x=20, y=32768) -> (x/y=w665:dbl)
                      n278 = Multiply(x=w665, y=w668) -> (x*y=w670:dbl)
                      n279 = Add(x=w663, y=w670) -> (x+y=w653:dbl)
                      n280 = Greater?(x=w662, y="Max Current") -> (0:w660:bool)
                      n281 = Select(t=4, s=w660, f=3) -> (s? t:f=w657:i32)
                      n282 = local write "Contact Cycles"(0) -> ()
                      n283 = Less?(x=w653, y=w655) -> (x < y?=w654:bool)
                      n284 = Select(t=w653, s=w654, f=w655) -> (s? t:f=w652:dbl)
                    }
                    frame 4 {
                      w672 = 0.0
                      w690 = 10
                      # "Make contact cycles after current saturation"
                      n285 = Divide(x=w673, y=15.13) -> (x/y=w686:dbl)
                      n286 = local read "Contact Cycles"() -> (w680:i32)
                      n287 = Divide(x=20, y=32768) -> (x/y=w676:dbl)
                      n288 = Multiply(x=w676, y=w686) -> (x*y=w688:dbl)
                      n289 = Add(x=w675, y=w688) -> (x+y=w677:dbl)
                      n290 = Increment(x=w680) -> (x+1=w679:i32)
                      n291 = Less?(x=w677, y=w690) -> (x < y?=w689:bool)
                      n292 = Select(t=w677, s=w689, f=w690) -> (s? t:f=w678:dbl)
                      n293 = Less Or Equal?(x="Make Contact", y=w679) -> (x <= y?=w683:bool)
                      n294 = local write "Contact Cycles"(w679) -> ()
                      n295 = Initialize Array(w672, w672) -> (w671:dbl[])
                      n296 = Select(t=1, s=w683, f=4) -> (s? t:f=w674:i32)
                    }
                  }
                  n297 = local write "Analog Output 1"(w589) -> ()
                  n298 = Build Array(w595, w589) -> ()  [unwired: 1 out]
                  n299 = call-poly <vilib>:"DAQmx Write.vi"("task/channels in"=w600, "auto start"=TRUE, "data"=w589, "error in"=w599) -> ("task out"=w598:refnum<k21>, "error out"=w597:errorcluster)  [unwired: 9 in, 1 out]
                }
              }
              "Case" <- w538
            }
            n300 = call <vilib>:"DAQmx Clear Task.vi"("task in"=w500, "error in"=w502) -> ("error out"=w501:errorcluster)  [unwired: 13 in]
            n301 = Not(x=w476) -> (.not. x?=w475:bool)
            n302 = call <vilib>:"DAQmx Clear Task.vi"("task in"=w505, "error in"=w504) -> ("error out"=w503:errorcluster)  [unwired: 13 in]
            n303 = local write "Tapping"(w475) -> ()
            n304 = Merge Errors(w503, w501) -> (w498:errorcluster)
            n305 = call <vilib>:"General Error Handler.vi"("type of dialog (OK msg:1)"=w499, "error in (no error)"=w498) -> ()  [unwired: 9 in, 5 out]
          }
          frame 8 {
            w697 = 0.0
            w711 = T2 3 items=["no dialog", "OK message", "continue or stop message", "OK message + warnings", "continue/stop + warnings"] ("type of dialog (OK msg:1)")
            w724 = 10123 items=["Finite Samples"=10178, "Continuous Samples"=10123] ("sample mode")
            w718 = 10123 items=["Finite Samples"=10178, "Continuous Samples"=10123] ("sample mode")
            n306 = call-poly <vilib>:"DAQmx Create Virtual Channel.vi"("maximum value"=10.0 ("maximum value 2"), "minimum value"=-10.0 ("minimum value 2"), "physical channels"=tag "Dev1/ao0:1" ("physical channels 2")) -> ("task out"=w725:refnum<k21>, "error out"=w726:errorcluster)  [unwired: 11 in]
            n307 = call-poly <vilib>:"DAQmx Create Virtual Channel.vi"("maximum value"=10.0 ("Maximum Value 2"), "minimum value"=-10.0 ("Minimum Value 2"), "physical channels"=tag "Dev1/ai0" ("Physical Channel 2")) -> ("task out"=w720:refnum<k21>, "error out"=w719:errorcluster)  [unwired: 11 in]
            n308 = call-poly <vilib>:"DAQmx Timing.vi"("task/channels in"=w725, "sample mode"=w724, "rate"=10000.0 ("rate 2"), "error in"=w726) -> ("task out"=w733:refnum<k21>, "error out"=w734:errorcluster)  [unwired: 10 in]
            n309 = call-poly <vilib>:"DAQmx Timing.vi"("task/channels in"=w720, "sample mode"=w718, "rate"=10000.0 ("Rate 2"), "error in"=w719) -> ("task out"=w736:refnum<k21>, "error out"=w737:errorcluster)  [unwired: 10 in]
            n310 = property class="DAQmx Timing" props=["Sample Clock:Rate"](reference=w733, error in=w734) -> (reference out=w732:refnum<k21>, error out=w735:errorcluster)  [unwired: 1 out]
            n311 = property class="DAQmx Timing" props=["Sample Clock:Rate"](reference=w736, error in=w737) -> (reference out=w738:refnum<k21>, error out=w739:errorcluster)  [unwired: 1 out]
            n312 = call "Get Terminal Name with Device Prefix.vi"("error in (no error)"=w739, "Local Terminal Name"="ai/StartTrigger" ("terminal"), "task/channels in"=w738) -> ("error out"=w709:errorcluster, "Terminal Name with Device Prefix"=w731:tag, "task out"=w707:refnum<k21>)  [unwired: 6 in]
            n313 = call-poly <vilib>:"DAQmx Trigger.vi"("task/channels in"=w732, "source"=w731, "error in"=w735) -> ("task out"=w705:refnum<k21>, "error out"=w702:errorcluster)  [unwired: 11 in]
            n314 = call <vilib>:"DAQmx Start Task.vi"("task/channels in"=w707, "error in"=w709) -> ("task out"=w706:refnum<k21>, "error out"=w708:errorcluster)  [unwired: 12 in]
            n315 = call <vilib>:"DAQmx Start Task.vi"("task/channels in"=w705, "error in"=w702) -> ("task out"=w704:refnum<k21>, "error out"=w703:errorcluster)  [unwired: 12 in]
            n316 = Initialize Array(w697, w697) -> ()  [unwired: 1 out]
            n317 = while {
              tunnel: w706 -> [w774]
              tunnel: w708 -> [w773]
              tunnel: w704 -> [w763]
              tunnel: w703 -> [w762]
              tunnel: [w772] -> w715
              tunnel: [w771] -> w714
              shift-right: [w748] -> w698
              shift-left: w701 -> [w753]
              tunnel: [w761] -> w696
              tunnel: [w760] -> w695
              tunnel: w692 -> [w744]
              i -> [w759]
              stop <- w749 stop-if-true
              w757 = 5e-05
              n318 = Absolute Value(x="Setpoint") -> (abs(x)=w740:dbl)
              n319 = call-poly <vilib>:"DAQmx Read.vi"("task/channels in"=w774, "error in"=w773) -> ("task out"=w772:refnum<k21>, "data"=w743:dbl, "error out"=w771:errorcluster)  [unwired: 11 in]
              n320 = Absolute Value(x=w743) -> (abs(x)=w742:dbl)
              n321 = local read "Bias Offset Correct"() -> (w745:dbl)
              n322 = Bundle("Proportional Gain"="Proportional Gain", "Integral Gain"="Integral Gain", "Differential Gain"="Differential Gain") -> (w764:T3)  [unwired: 1 in]
              n323 = local write "Waveform Chart"(w743) -> ()
              n324 = Bundle(10, -10) -> (w768:cluster{i32, i32})  [unwired: 1 in]
              n325 = call-poly "PID.vi"("output range"=w768, "dt (s)"=w757, "PID gains"=w764, "process variable"=w742, "setpoint"=w740) -> ("output"=w756:dbl)  [unwired: 5 in, 1 out]
              n326 = Add(x=w744, y=w745) -> (x+y=w746:dbl)
              n327 = Less?(x=w759, y=1000) -> (x < y?=w754:bool)
              n328 = call-poly "PID Output Rate Limiter.vi"("reinitialize? (F)"=w754, "dt (s)"=w757, "output rate (EGU/min)"="Piezo Delta rate", "initial output"=w753, "input (controller output)"=w756) -> ("output"=w748:dbl)  [unwired: 3 in, 1 out]
              n329 = local write "Analog Output 1"(w748) -> ()
              n330 = Build Array(w746, w748) -> (w747:dbl[])
              n331 = local read "Sweep Bias"() -> (w752:bool)
              n332 = local read "PID"() -> (w750:bool)
              n333 = call-poly <vilib>:"DAQmx Write.vi"("task/channels in"=w763, "data"=w747, "error in"=w762) -> ("task out"=w761:refnum<k21>, "error out"=w760:errorcluster)  [unwired: 10 in, 1 out]
              n334 = Not(x=w750) -> (.not. x?=w751:bool)
              n335 = Compound Arithmetic op=OR(w752, w751) -> (w749:bool)
            }
            n336 = call <vilib>:"DAQmx Clear Task.vi"("task in"=w696, "error in"=w695) -> ("error out"=w712:errorcluster)  [unwired: 13 in]
            n337 = call <vilib>:"DAQmx Clear Task.vi"("task in"=w715, "error in"=w714) -> ("error out"=w713:errorcluster)  [unwired: 13 in]
            n338 = Merge Errors(w713, w712) -> (w710:errorcluster)
            n339 = call <vilib>:"General Error Handler.vi"("type of dialog (OK msg:1)"=w711, "error in (no error)"=w710) -> ()  [unwired: 9 in, 5 out]
          }
        }
      }
    }
  }
